vi "Test - All-In-One (SubVI).vi"(0 "START TEST":bool, 1 "STOP TEST":bool, 2 "NEXT STEP":bool, 3 "HOLD STEP":bool, 4 "Test Folder":path, 5 "Error Input":errorcluster, 7 "Test Cluster":T2={"Load Test"=0, "New Test Name"="", "Test Description"="", "Step Select"=0, "Save Test"=FALSE, "Erase Test"=FALSE, "Max Steps"=15, "Loop Limit"=5, "Continue at Loop Limit?"=FALSE, "Step N"=2, "Test Array (Standard)"=[{"Step Number"=0, "Step Description"="Step Description", "Step Time Target"=10.0, "Step Time Unit"=0, "Step End Action"=0}], "Test Array (Custom)"=[{"Custom Actions"=0, "ch0"=FALSE, "ch1"=FALSE, "ch2"=FALSE, "ch3"=FALSE}]} {"Test Array (Custom)"."Custom Actions" items=["None", "Measure Signal", "Display Plot", "Save to File"]; "Test Array (Standard)"."Step End Action" items=["Go to Next Step", "Loop to Step 0", "Loop to Step N", "Stop Test Mode", "Stop Program"]; "Test Array (Standard)"."Step Time Unit" items=["sec", "min", "hr"]; "Test Array (Standard)"."Step Time Target" min=0.01 format="%#.2f"; "Test Array (Standard)"."Step Number" min=0 step=1; "Load Test" items=["123", "a", "b", "c"]; "Step Select" step=1}, 9 "Test Cluster Ref":refnum<vi>) -> (11 "Stop Program?":bool, 13 "Test Running?":bool, 14 "Test Display":string="Mode: OFF  (Press Start to Begin)\r\r\r    ", 15 "Test Output":T1, 16 "Step Complete?":bool=TRUE, 17 "Step Number":u16, 18 "Loop Number":u16, 19 "Error Output":errorcluster)   [LabVIEW 2012]
panel:
  # "NOTE:  The only things that should need to be modified\nfor a different program are highlighted in green (on block diagram)!"
  # "9481 Relay"
  # "Custom Action"
  # "Scroll"
  # "Step"
  # "Description"
  # "Time Target"
  # "End Action"
  # "0"
  # "1"
  # "2"
  # "3"
  # "Total #\nof Steps"
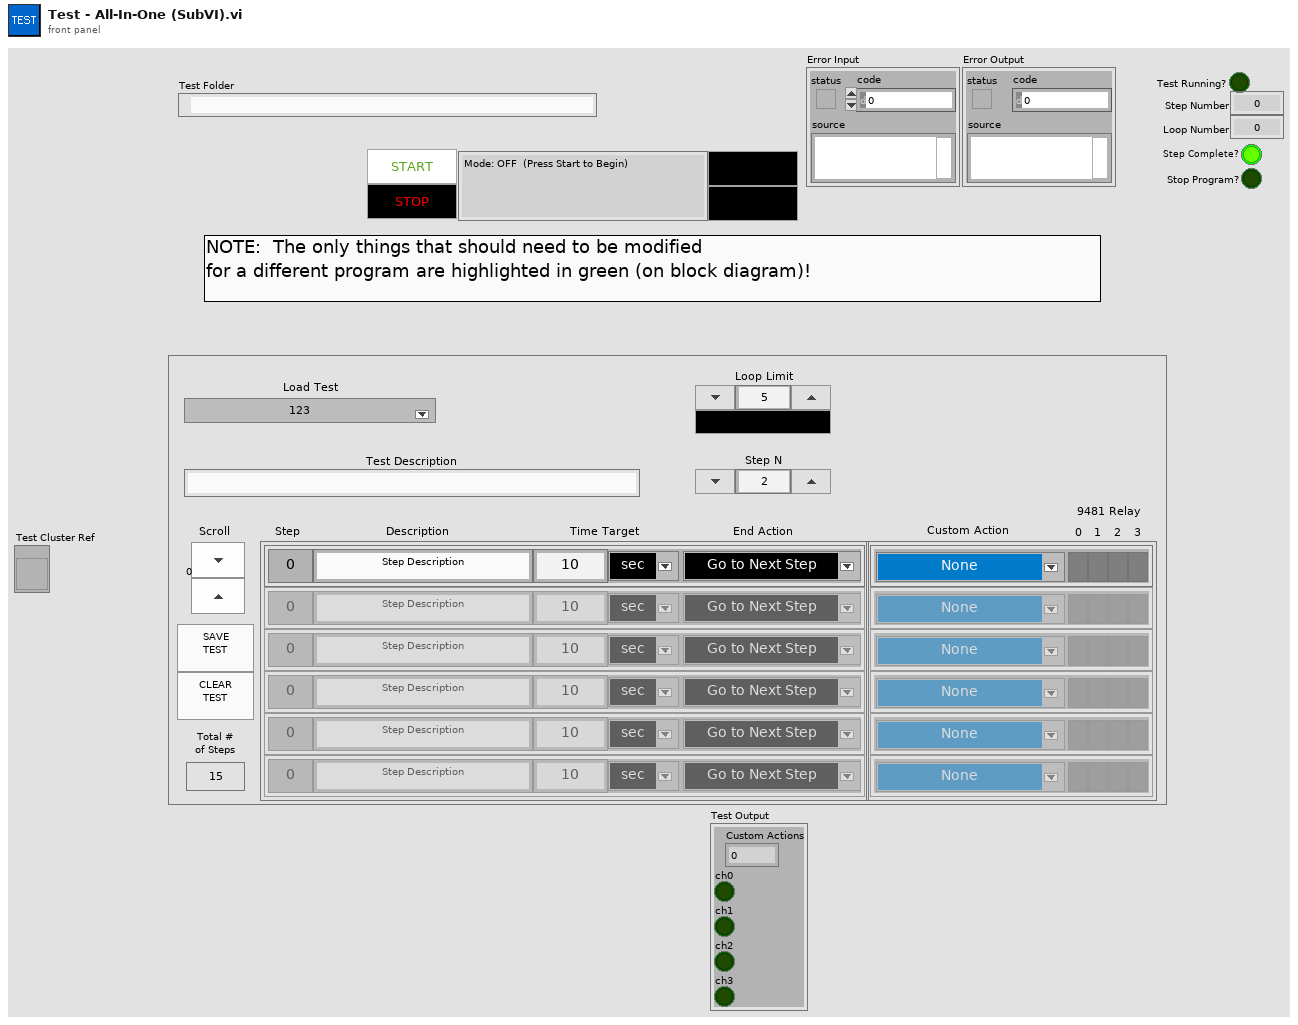
[diagram p1: front panel]
types:
  T1 = cluster{"Custom Actions":u16, "ch0":bool, "ch1":bool, "ch2":bool, "ch3":bool}
  T2 = cluster{"Load Test":u16, "New Test Name":string, "Test Description":string, "Step Select":u16, "Save Test":bool, "Erase Test":bool, "Max Steps":u16, "Loop Limit":u16, "Continue at Loop Limit?":bool, "Step N":u16, "Test Array (Standard)":cluster{"Step Number":i32, "Step Description":string, "Step Time Target":dbl, "Step Time Unit":u16, "Step End Action":u16}[], "Test Array (Custom)":cluster{"Custom Actions":u16, "ch0":bool, "ch1":bool, "ch2":bool, "ch3":bool}[]}
  T3 = cluster{"Load Test Ring":i32, "New Test Name":i32, "Test Description":i32, "Step Select":i32, "Save Test":i32, "Erase Test":i32, "Max Steps":i32, "Loop Limit":i32, "Continue at Loop Limit":i32, "Step N":i32, "Test Array (Standard)":i32, "Test Array (Custom)":i32}
  T4 = enum8{"Enabled", "Disabled", "Disabled and Grayed Out"}
  T5 = cluster{"Step Number":i32, "Step Description":string, "Step Time Target":dbl, "Step Time Unit":u16, "Step End Action":u16}[]
  T6 = cluster{"Custom Actions":u16, "ch0":bool, "ch1":bool, "ch2":bool, "ch3":bool}[]
  T7 = enum16{"open", "replace", "create", "open or create", "replace or create", "replace or create with confirmation"}
  T8 = cluster{"Step Number":i32, "Step Description":string, "Step Time Target":dbl, "Step Time Unit":u16, "Step End Action":u16}
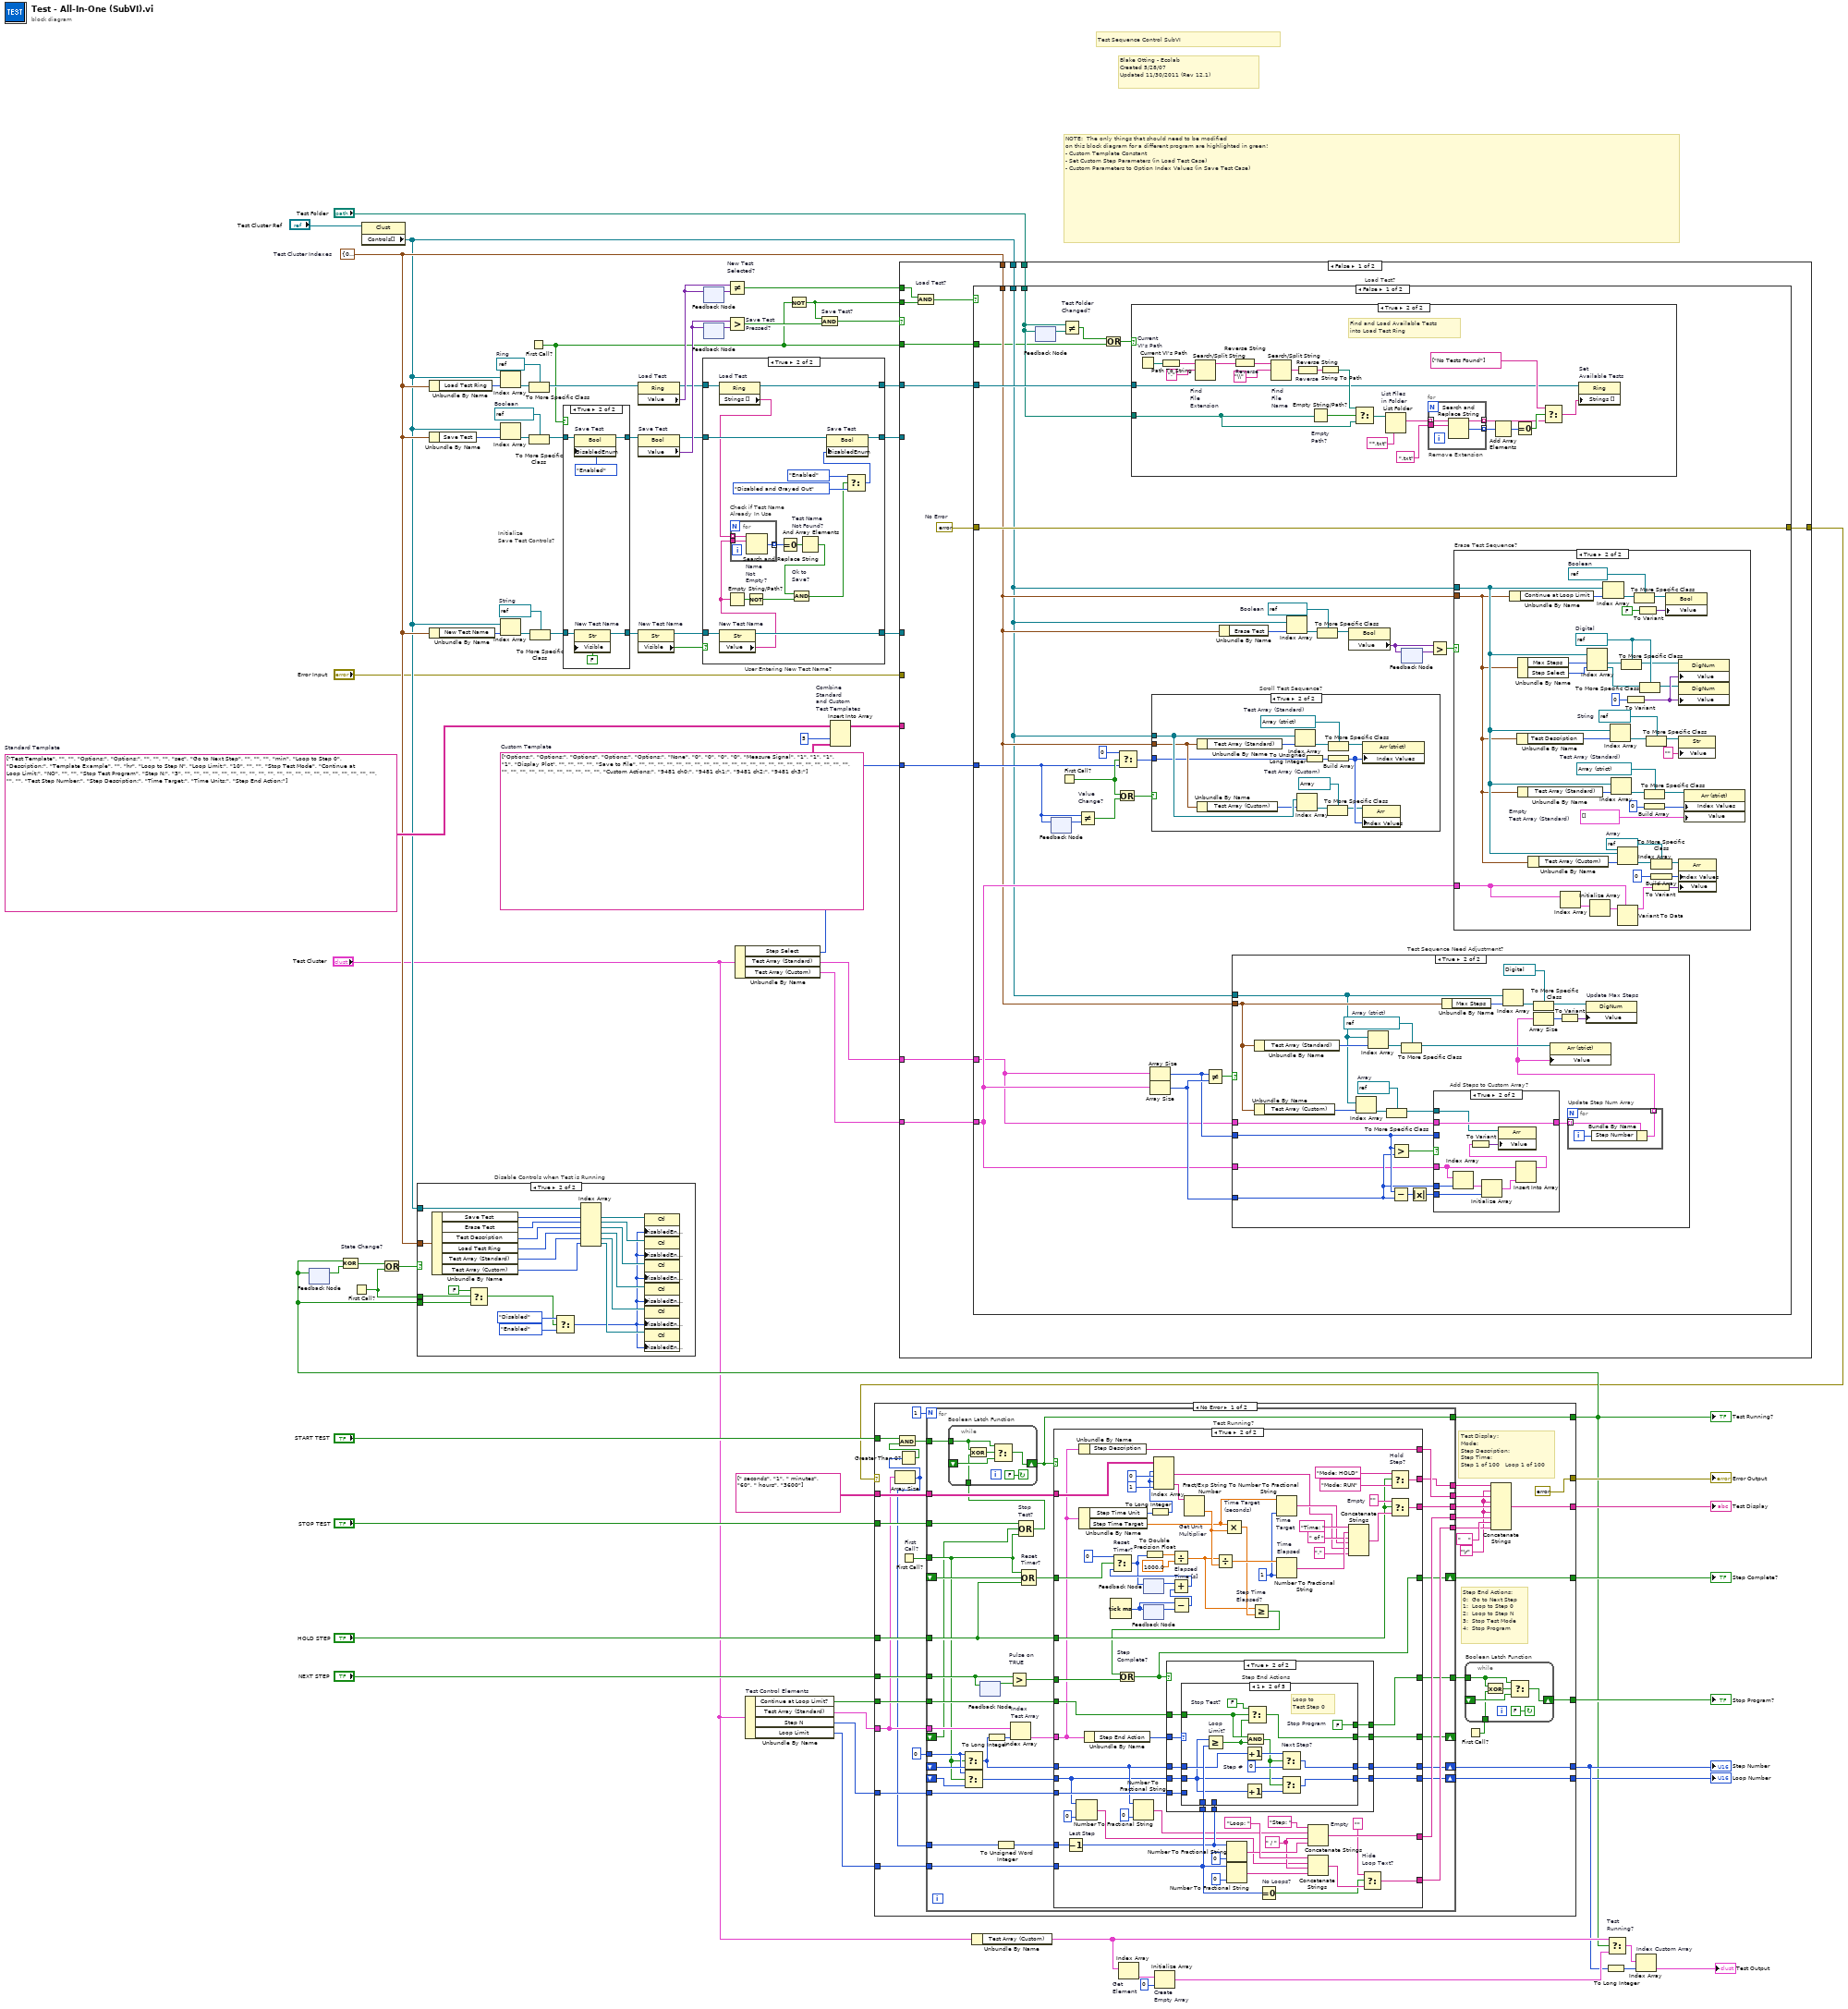
[diagram p0: block diagram]
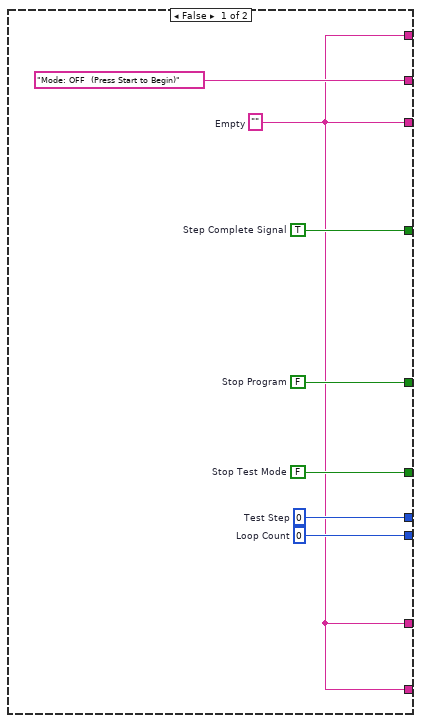
[diagram p3: hidden frame]
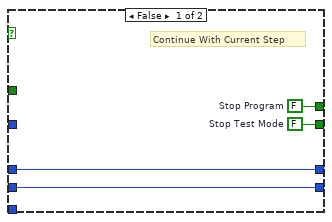
[diagram p4: hidden frame]
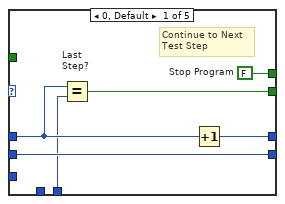
[diagram p5: hidden frame]
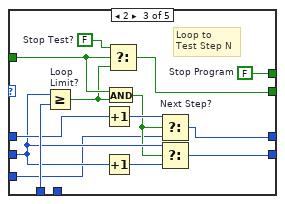
[diagram p6: hidden frame]
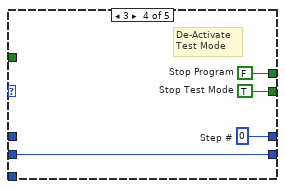
[diagram p7: hidden frame]
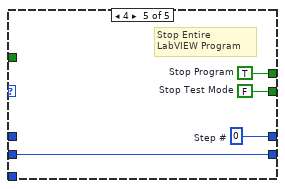
[diagram p8: hidden frame]
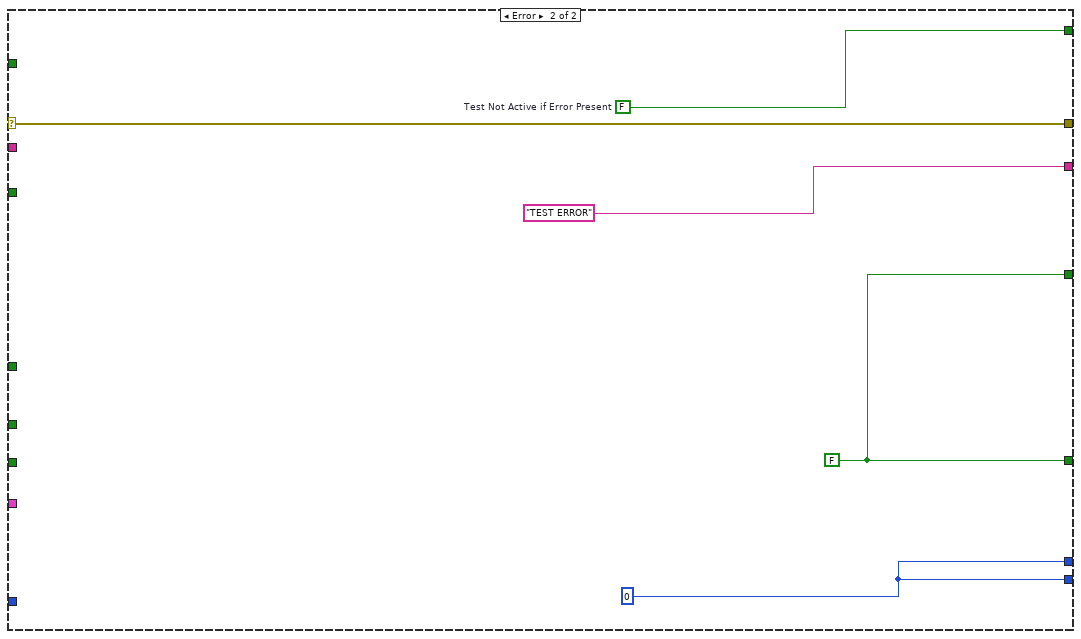
[diagram p9: hidden frame]
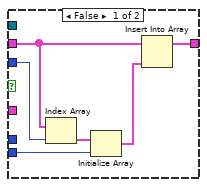
[diagram p13: hidden frame]
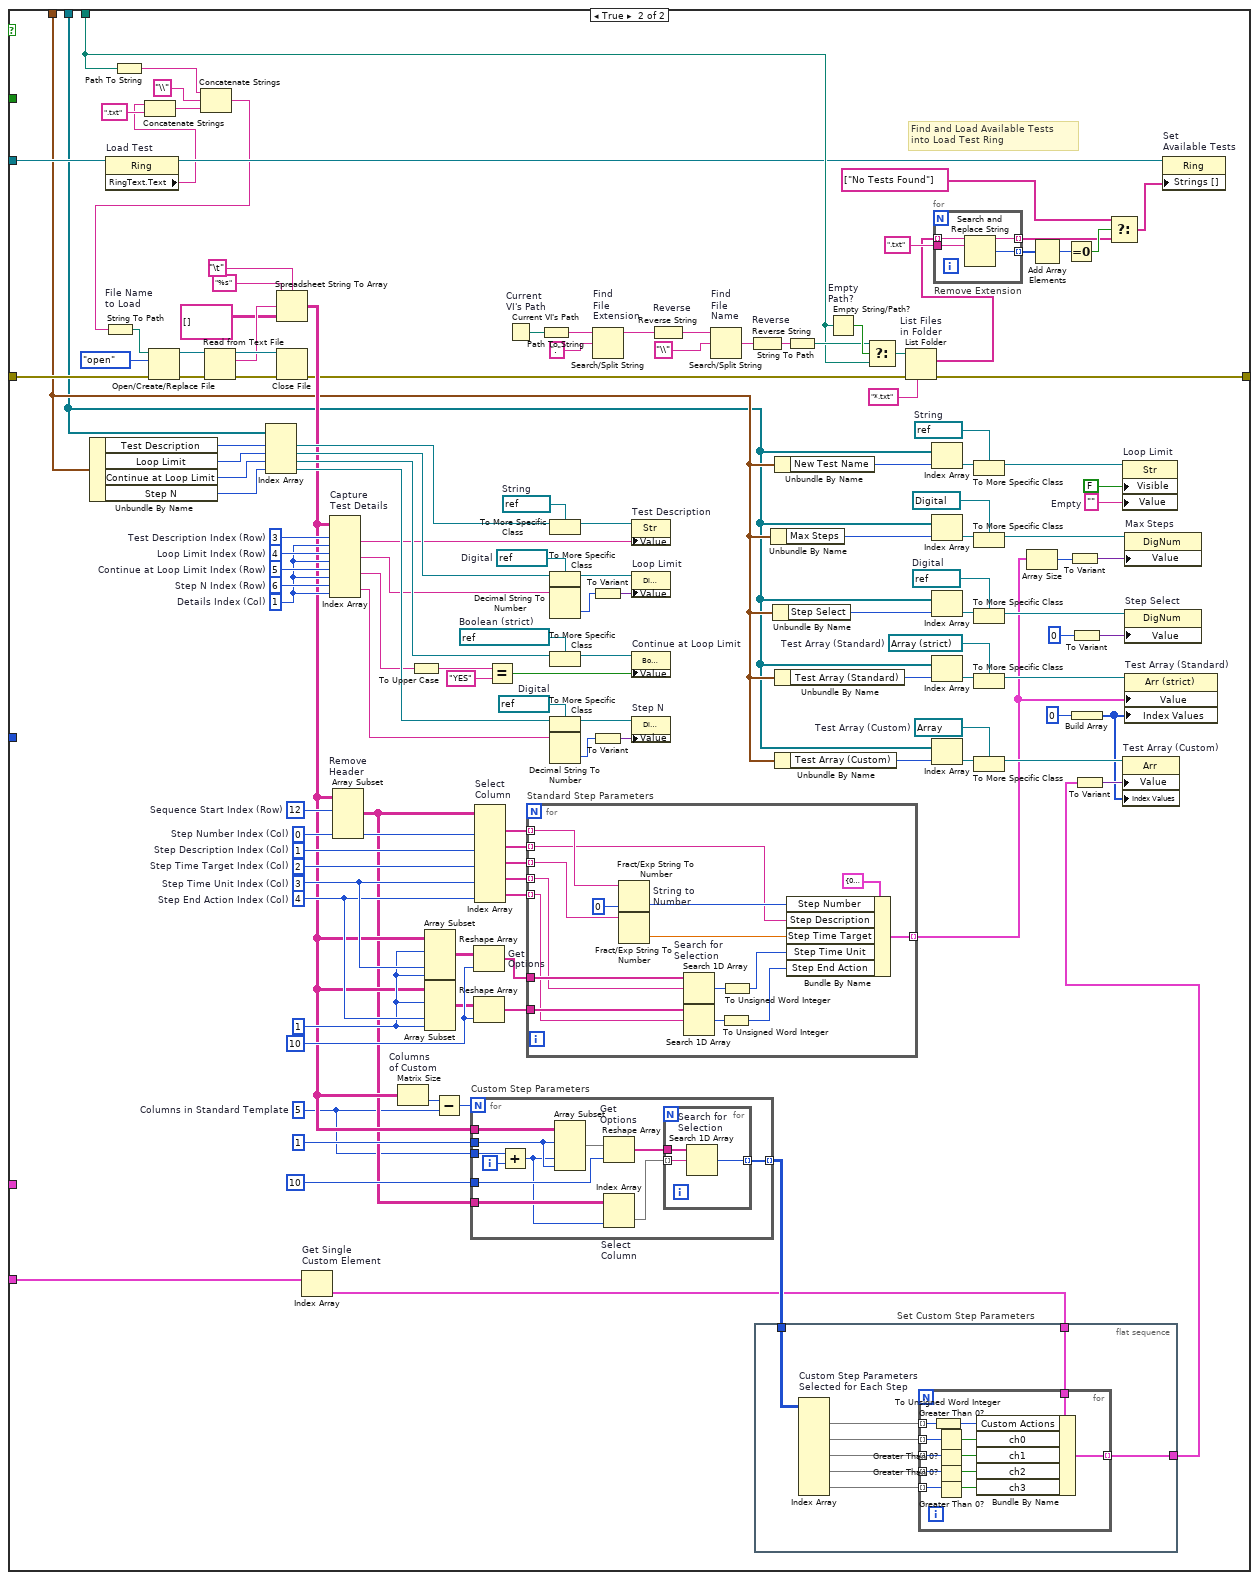
[diagram p17: hidden frame]
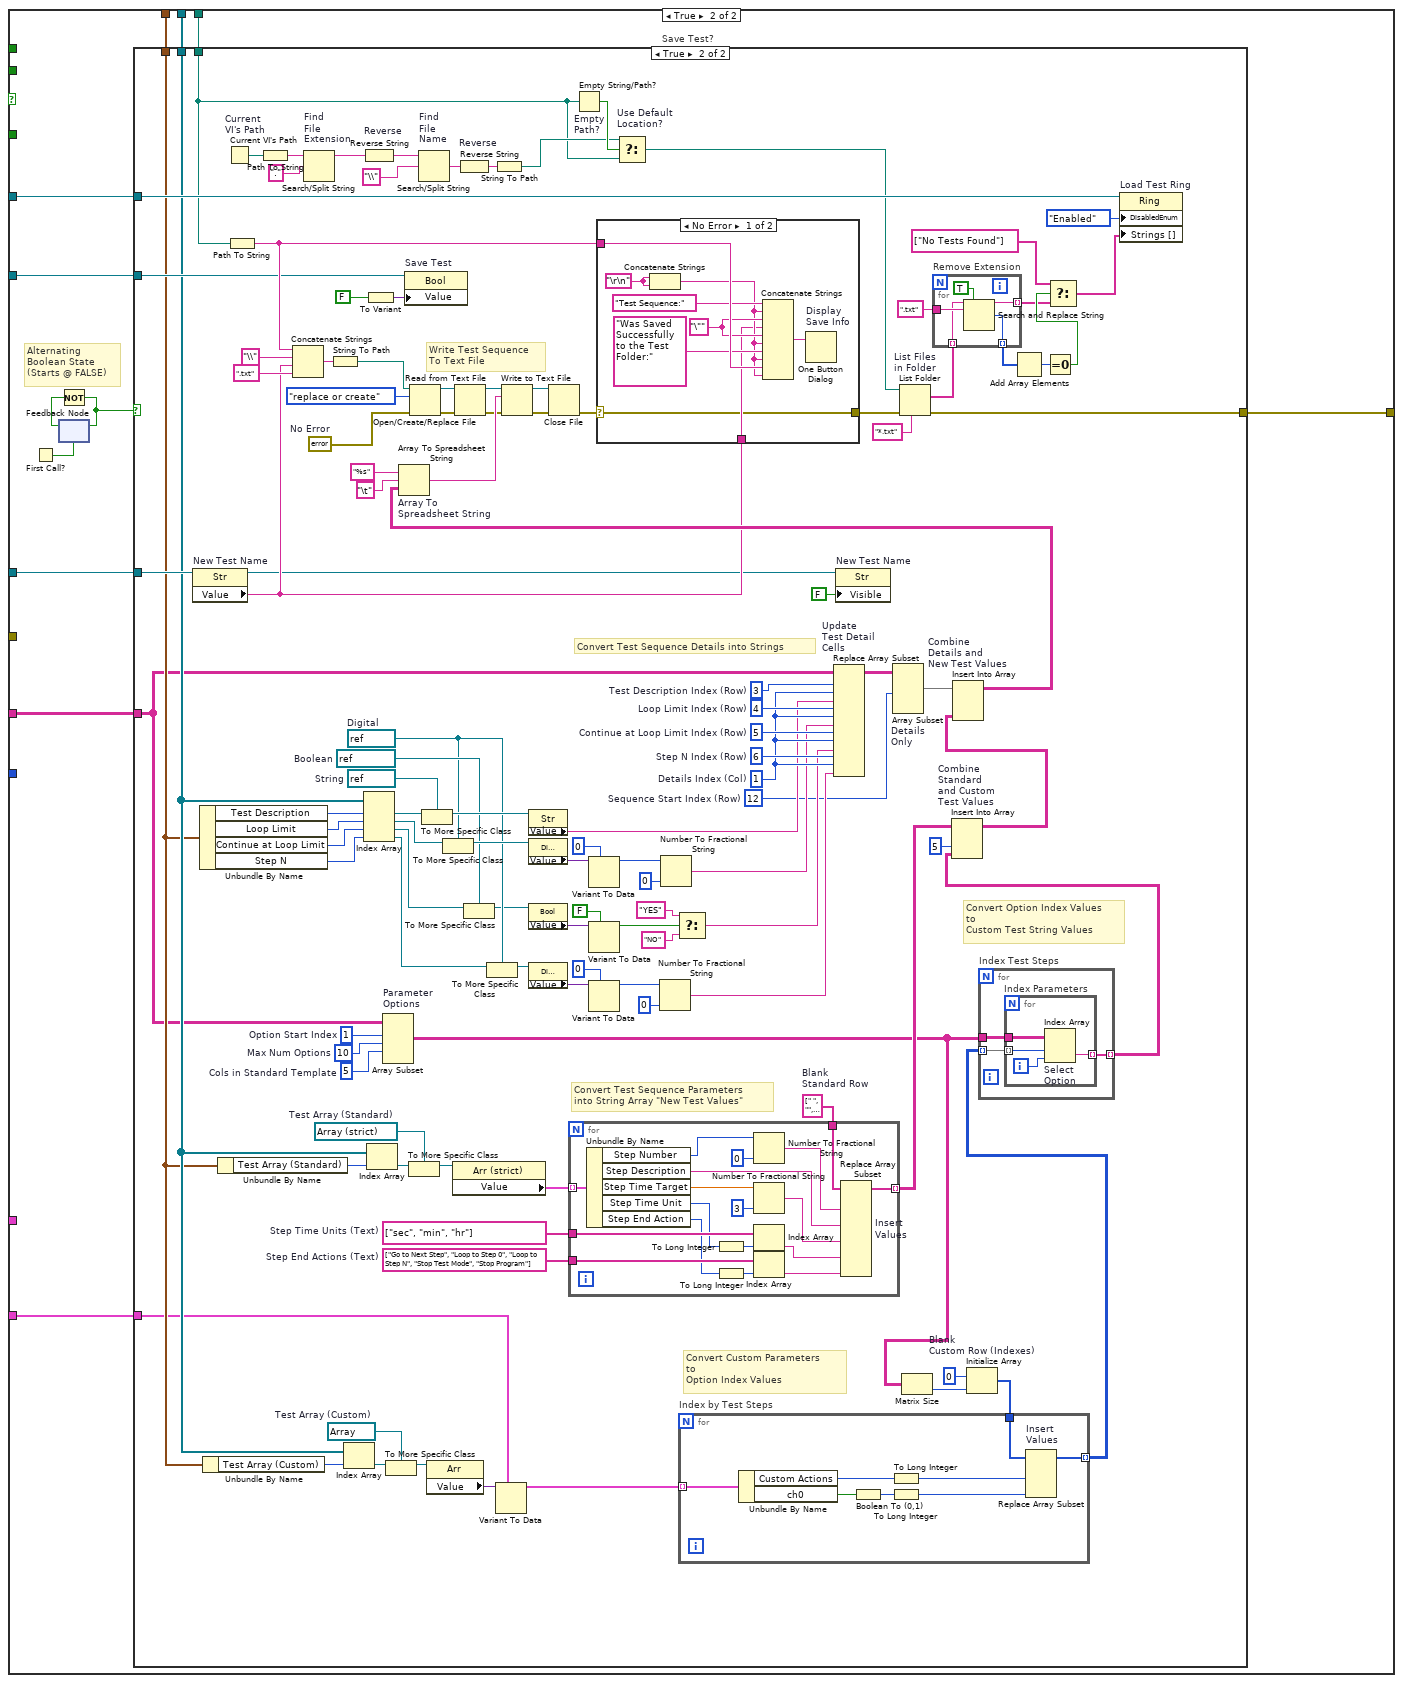
[diagram p18: hidden frame]
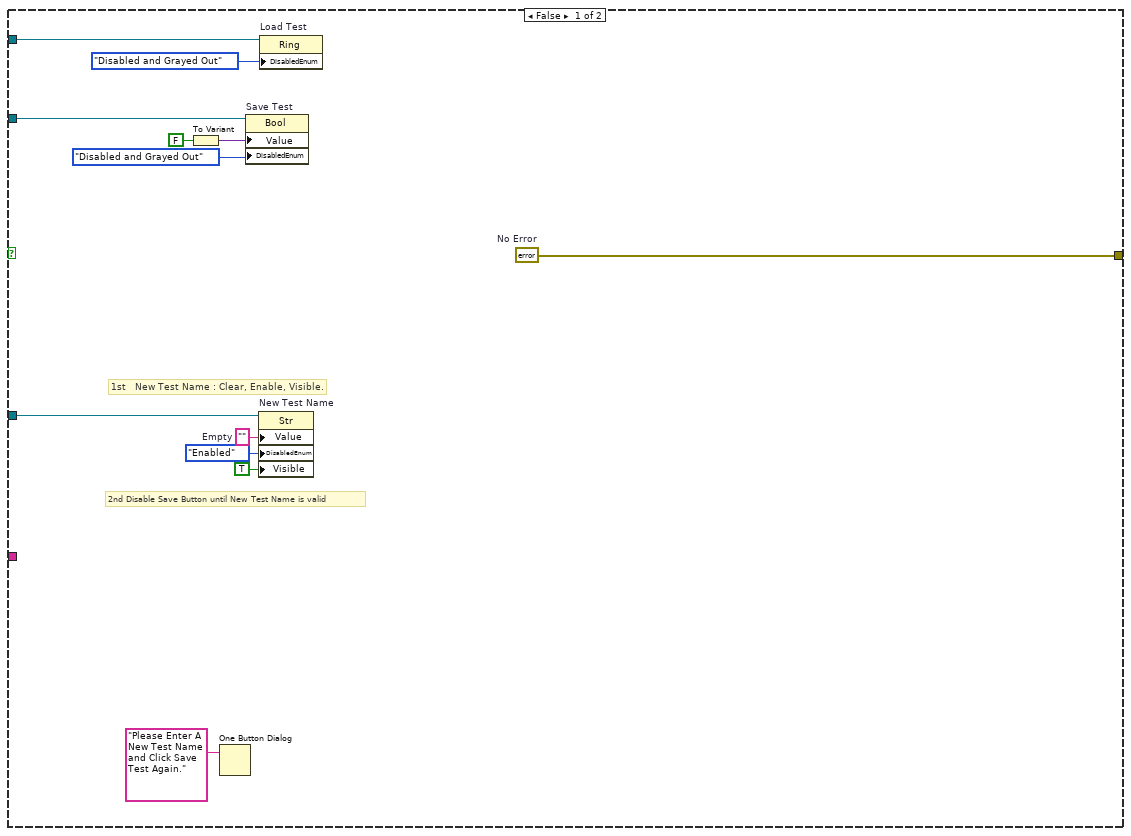
[diagram p19: hidden frame]
diagram:
  w33 = refnum<vi> refnum  # Ring
  w55 = refnum<vi> refnum  # Boolean
  w59 = refnum<vi> refnum  # String
  w64 = string[][] [["Options:", "Options:", "Options", "Options:", "Options:"], ["None", "0", "0", "0", "0"], ["Measure Signal", "1", "1", "1", "1"], ["Display Plot", "", "", "", ""], ["Save to File", "", "", "", ""], ["", "", "", "", ""], ["", "", "", "", ""], ["", "", "", "", ""], ["", "", "", "", ""], ["", "", "", "", ""], ["", "", "", "", ""], ["Custom Actions:", "9481 ch0:", "9481 ch1:", "9481 ch2:", "9481 ch3:"]]  # Custom Template
  w66 = T3 {"Load Test Ring"=0, "New Test Name"=1, "Test Description"=2, "Step Select"=3, "Save Test"=4, "Erase Test"=5, "Max Steps"=6, "Loop Limit"=7, "Continue at Loop Limit"=8, "Step N"=9, "Test Array (Standard)"=10, "Test Array (Custom)"=11}  # Test Cluster Indexes
  w71 = string[][] [["Test Template", "", "", "Options:", "Options:"], ["", "", "", "sec", "Go to Next Step"], ["", "", "", "min", "Loop to Step 0"], ["Description:", "Template Example", "", "hr", "Loop to Step N"], ["Loop Limit:", "10", "", "", "Stop Test Mode"], ["Continue at Loop Limit:", "NO", "", "", "Stop Test Program"], ["Step N:", "3", "", "", ""], ["", "", "", "", ""], ["", "", "", "", ""], ["", "", "", "", ""], ["", "", "", "", ""], ["Test Step Number:", "Step Description:", "Time Target:", "Time Units:", "Step End Action:"]]  # Standard Template
  # "NOTE:  The only things that should need to be modified\non this block diagram for a different program are highlighted in green!\n- Custom Template Constant\n- Set Custom Step Parameters (in Load Test Case)\n- Custom Parameters to Option Index Values (in Save Test Case)"
  # "Blake Otting - Ecolab\nCreated 5/28/07\nUpdated 11/30/2011 (Rev 12.1)"
  # "Test Sequence Control SubVI"
  n1 = feedback #1() -> (w30:bool)  [unwired: 1 in]
  n2 = First Call?() -> (First Call?: T/F=w27:bool)
  n3 = property class="Clust"(reference="Test Cluster Ref") -> ("Controls[]"=w65:refnum<vi>[])  [unwired: 1 in, 2 out]
  n4 = Unbundle By Name(w66) -> ("Load Test Ring"=w34:i32)
  n5 = Unbundle By Name(w66) -> ("Save Test"=w57:i32)
  n6 = Unbundle By Name(w66) -> ("New Test Name"=w61:i32)
  n7 = Index Array(array=w65, index=w34) -> (element=w32:refnum<vi>)
  n8 = Index Array(array=w65, index=w57) -> (element=w56:refnum<vi>)
  n9 = Index Array(array=w65, index=w61) -> (element=w60:refnum<vi>)
  n10 = First Call?() -> (First Call?: T/F=w8:bool)
  n11 = To More Specific Class(target class=w33, reference=w32) -> (specific class reference=w31:refnum<vi>)  [unwired: 1 in, 1 out]
  n12 = To More Specific Class(target class=w55, reference=w56) -> (specific class reference=w44:refnum<vi>)  [unwired: 1 in, 1 out]
  n13 = To More Specific Class(target class=w59, reference=w60) -> (specific class reference=w46:refnum<vi>)  [unwired: 1 in, 1 out]
  n14 = case "Initialize\nSave Test Controls?" shown="True" w8 {
    tunnel: w44 -> [w72 w79]
    tunnel: [w72 w78] -> w43
    tunnel: w46 -> [w73 w77]
    tunnel: [w73 w76] -> w45
    frame False {
    }
    frame True {
      n15 = property on="Save Test" class="Bool"(reference=w79, "DisabledEnum"=T4."Enabled" ("Disabled")) -> (reference out=w78:refnum<vi>)  [unwired: 1 in, 1 out]
      n16 = property on="New Test Name" class="Str"(reference=w77, "Visible"=FALSE) -> (reference out=w76:refnum<vi>)  [unwired: 1 in, 1 out]
    }
  }
  n17 = property on="Load Test" class="Ring"(reference=w31) -> (reference out=w39:refnum<vi>, "Value"=w40:variant)  [unwired: 1 in, 1 out]
  n18 = property on="Save Test" class="Bool"(reference=w43) -> (reference out=w49:refnum<vi>, "Value"=w53:variant)  [unwired: 1 in, 1 out]
  n19 = property on="New Test Name" class="Str"(reference=w45) -> (reference out=w51:refnum<vi>, "Visible"=w52:bool)  [unwired: 1 in, 1 out]
  n20 = case "User Entering New Test Name?" shown="True" w52 {
    tunnel: w51 -> [w82 w95]
    tunnel: w39 -> [w81 w94]
    tunnel: [w82 w90] -> w48
    tunnel: [w81 w89] -> w50
    tunnel: w49 -> [w80 w88]
    tunnel: [w80 w87] -> w47
    frame False {
    }
    frame True {
      n21 = property on="Load Test" class="Ring"(reference=w94) -> (reference out=w89:refnum<vi>, "Strings []"=w84:string[])  [unwired: 1 in, 1 out]
      n22 = property on="New Test Name" class="Str"(reference=w95) -> (reference out=w90:refnum<vi>, "Value"=w83:string)  [unwired: 1 in, 1 out]
      n23 = Empty String/Path?(string/path=w83) -> (empty?=w96:bool)
      n24 = for "Check if Test Name\nAlready In Use" {
        tunnel: w84 -> [w102] mode=indexing
        tunnel: w83 -> [w101]
        tunnel: [w100] -> w99 mode=indexing
        n25 = Search and Replace String(input string=w102, search string=w101) -> (number of replacements=w100:i32)  [unwired: 6 in, 3 out]
      }
      n26 = Not "Name\nNot\nEmpty?"(x=w96) -> (.not. x?=w91:bool)
      n27 = Equal To 0?(x=w99) -> (x = 0?=w98:bool[])
      n28 = And Array Elements "Test Name\nNot Found?"(Boolean array=w98) -> (logical AND=w97:bool)
      n29 = And "Ok to\nSave?"(x=w97, y=w91) -> (x .and. y?=w85:bool)
      n30 = Select(t=T4."Enabled" ("Disabled"), s=w85, f=T4."Disabled and Grayed Out" ("Disabled")) -> (s? t:f=w86:T4)
      n31 = property on="Save Test" class="Bool"(reference=w88, "DisabledEnum"=w86) -> (reference out=w87:refnum<vi>)  [unwired: 1 in, 1 out]
    }
  }
  n32 = feedback #2() -> (w41:variant)  [unwired: 1 in]
  n33 = feedback-in #2(w40) -> ()
  n34 = feedback #3() -> (w54:variant)  [unwired: 1 in]
  n35 = feedback-in #3(w53) -> ()
  n36 = Not Equal? "New Test\nSelected?"(x=w40, y=w41) -> (x != y?=w4:bool)
  n37 = Greater? "Save Test\nPressed?"(x=w53, y=w54) -> (0:w38:bool)
  n38 = Unbundle By Name("Test Cluster") -> ("Step Select"=w21:u16, "Test Array (Standard)"=w23:T5, "Test Array (Custom)"=w22:T6)
  n39 = Unbundle By Name "Test Control Elements"("Test Cluster") -> ("Continue at Loop Limit?"=w26:bool, "Test Array (Standard)"=w6:T5, "Step N"=w25:u16, "Loop Limit"=w24:u16)
  n40 = Not(x=w8) -> (.not. x?=w37:bool)
  n41 = And "Save Test?"(x=w37, y=w38) -> (x .and. y?=w42:bool)
  n42 = Insert Into Array "Combine\nStandard\nand Custom\nTest Templates"(array=w71, index (col)=5 ("disabled index (col)"), new element=w64) -> (w58:string[][])  [unwired: 1 in]
  n43 = case shown="False" w42 {
    tunnel: "Test Folder" -> [w111 w455]
    tunnel: w22 -> [w112 w456]
    tunnel: w58 -> [_ w457]
    tunnel: w66 -> [w114 w461]
    tunnel: w65 -> [w115 w462]
    tunnel: w47 -> [_ w460]
    tunnel: w48 -> [_ w459]
    tunnel: w50 -> [w113 w458]
    tunnel: [w106 w454] -> w7
    tunnel: "Error Input" -> [_ _]
    tunnel: w4 -> [w108 _]
    tunnel: w8 -> [w110 _]
    tunnel: w37 -> [w107 _]
    tunnel: w21 -> [w105 _]
    tunnel: w23 -> [w104 _]
    frame False {
      w103 = errorcluster {"status"=FALSE, "code"=0, "source"=""}  # No Error
      n44 = And "Load Test?"(x=w108, y=w107) -> (x .and. y?=w109:bool)
      n45 = case "Load Test?" shown="False" w109 {
        tunnel: w115 -> [w122 w267]
        tunnel: w114 -> [w123 w268]
        tunnel: w112 -> [w124 w399]
        tunnel: [w143 w276] -> w106
        tunnel: w103 -> [w143 w269]
        tunnel: w113 -> [w142 w273]
        tunnel: w110 -> [w117 _]
        tunnel: w111 -> [w119 w274]
        tunnel: w105 -> [w135 _]
        tunnel: w104 -> [w121 _]
        frame False {
          w130 = refnum<vi> refnum  # Boolean
          n46 = feedback #4() -> (w120:path)  [unwired: 1 in]
          n47 = feedback-in #4(w119) -> ()
          n48 = feedback #5() -> (w136:u16)  [unwired: 1 in]
          n49 = feedback-in #5(w135) -> ()
          n50 = First Call?() -> (First Call?: T/F=w140:bool)
          n51 = Not Equal? "Test Folder\nChanged?"(x=w119, y=w120) -> (x != y?=w118:bool)
          n52 = Not Equal? "Value\nChange?"(x=w135, y=w136) -> (x != y?=w137:bool)
          n53 = Or(x=w118, y=w117) -> (x .or. y?=w116:bool)
          n54 = Or(x=w140, y=w137) -> (x .or. y?=w138:bool)
          n55 = Select(t=u16 0 ("upper limit"), s=w140, f=w135) -> (s? t:f=w141:u16)
          n56 = case shown="True" w116 {
            tunnel: w142 -> [_ w241]
            tunnel: w119 -> [_ w240]
            frame False {
            }
            frame True {
              # "Find and Load Available Tests \ninto Load Test Ring"
              n57 = Current VI's Path "Current\nVI's Path"() -> (path=w251:path)
              n58 = Path To String(path=w251) -> (string=w256:string)
              n59 = Search/Split String "Find\nFile \nExtension"(string=w256, search string/char (-)=".") -> (substring before match=w255:string)  [unwired: 1 in, 2 out]
              n60 = Reverse String "Reverse"(1:w255) -> (0:w254:string)
              n61 = Search/Split String "Find\nFile \nName"(string=w254, search string/char (-)="\\") -> (match + rest of string=w252:string)  [unwired: 1 in, 2 out]
              n62 = Reverse String "Reverse"(1:w252) -> (0:w258:string)
              n63 = Empty String/Path? "Empty\nPath?"(string/path=w240) -> (empty?=w250:bool)
              n64 = String To Path(string=w258) -> (path=w249:path)
              n65 = Select(t=w249, s=w250, f=w240) -> (s? t:f=w259:path)
              n66 = List Folder "List Files\nin Folder"(path=w259, pattern="*.txt") -> (filenames=w261:string[])  [unwired: 1 in, 4 out]
              n67 = for "Remove Extension" {
                tunnel: w261 -> [w264] mode=indexing
                tunnel: ".txt" ("pattern") -> [w265]
                tunnel: [w263] -> w242 mode=indexing
                tunnel: [w262] -> w247 mode=indexing
                n68 = Search and Replace String(input string=w264, search string=w265) -> (result string=w263:string, number of replacements=w262:i32)  [unwired: 6 in, 2 out]
              }
              n69 = Add Array Elements(numeric array=w247) -> (sum=w246:i32)
              n70 = Equal To 0?(x=w246) -> (x = 0?=w245:bool)
              n71 = Select(t=string[] ["No Tests Found"], s=w245, f=w242) -> (s? t:f=w244:string[])
              n72 = property on="Set\nAvailable Tests" class="Ring"(reference=w241, "Strings []"=w244) -> ()  [unwired: 1 in, 2 out]
            }
          }
          n73 = Array Size(array=w121) -> (size(s)=w125:i32)
          n74 = Array Size(array=w124) -> (size(s)=w126:i32)
          n75 = case "Scroll Test Sequence?" shown="True" w138 {
            tunnel: w122 -> [_ w239]
            tunnel: w123 -> [_ w238]
            tunnel: w141 -> [_ w227]
            frame False {
            }
            frame True {
              w237 = refnum<vi> refnum  # Test Array (Custom)
              w234 = refnum<vi> refnum  # Test Array (Standard)
              n76 = Unbundle By Name(w238) -> ("Test Array (Standard)"=w235:i32)
              n77 = Unbundle By Name(w238) -> ("Test Array (Custom)"=w236:i32)
              n78 = Index Array(array=w239, index=w235) -> (element=w228:refnum<vi>)
              n79 = Index Array(array=w239, index=w236) -> (element=w231:refnum<vi>)
              n80 = To Unsigned Long Integer(number=w227) -> (unsigned 32bit integer=w230:u32)
              n81 = To More Specific Class(target class=w237, reference=w231) -> (specific class reference=w232:refnum<vi>)  [unwired: 1 in, 1 out]
              n82 = To More Specific Class(target class=w234, reference=w228) -> (specific class reference=w229:refnum<vi>)  [unwired: 1 in, 1 out]
              n83 = Build Array(w230) -> (w233:u32[])
              n84 = property class="Arr (strict)"(reference=w229, "Index Values"=w233) -> ()  [unwired: 1 in, 2 out]
              n85 = property class="Arr"(reference=w232, "Index Values"=w233) -> ()  [unwired: 1 in, 2 out]
            }
          }
          n86 = Not Equal?(x=w125, y=w126) -> (x != y?=w127:bool)
          n87 = Unbundle By Name(w123) -> ("Erase Test"=w128:i32)
          n88 = case "Test Sequence Need Adjustment?" shown="True" w127 {
            tunnel: w123 -> [_ w152]
            tunnel: w122 -> [_ w151]
            tunnel: w125 -> [_ w150]
            tunnel: w121 -> [_ w149]
            tunnel: w126 -> [_ w148]
            tunnel: w124 -> [_ w147]
            frame False {
            }
            frame True {
              w164 = refnum<vi> refnum  # Array
              w161 = refnum<vi> refnum  # Array (strict)
              n89 = Unbundle By Name(w152) -> ("Test Array (Standard)"=w162:i32)
              n90 = Unbundle By Name(w152) -> ("Test Array (Custom)"=w163:i32)
              n91 = Index Array(array=w151, index=w163) -> (element=w160:refnum<vi>)
              n92 = Index Array(array=w151, index=w162) -> (element=w159:refnum<vi>)
              n93 = To More Specific Class(target class=w164, reference=w160) -> (specific class reference=w146:refnum<vi>)  [unwired: 1 in, 1 out]
              n94 = Subtract(x=w150, y=w148) -> (x-y=w167:i32)
              n95 = Greater?(x=w150, y=w148) -> (0:w166:bool)
              n96 = To More Specific Class(target class=w161, reference=w159) -> (specific class reference=w145:refnum<vi>)  [unwired: 1 in, 1 out]
              n97 = Absolute Value(x=w167) -> (abs(x)=w168:i32)
              n98 = case "Add Steps to Custom Array?" shown="True" w166 {
                tunnel: w146 -> [_ w175]
                tunnel: w148 -> [_ w176]
                tunnel: w147 -> [_ w182]
                tunnel: w149 -> [w170 w177]
                tunnel: w168 -> [w174 w178]
                tunnel: w150 -> [w173 _]
                tunnel: [w169 w177] -> w165
                frame False {
                  n99 = Index Array(array=w170, index=w173) -> (element=w172:T8)
                  n100 = Initialize Array(w172, w174) -> (w171:T5)
                  n101 = Insert Into Array(array=w170, new element=w171) -> (w169:T5)  [unwired: 1 in]
                }
                frame True {
                  n102 = Index Array(array=w182, index=w176) -> (element=w183:T1)
                  n103 = Initialize Array(w183, w178) -> (w181:T6)
                  n104 = Insert Into Array(array=w182, new element=w181) -> (w180:T6)  [unwired: 1 in]
                  n105 = To Variant(anything=w180) -> (Variant=w179:variant)
                  n106 = property class="Arr"(reference=w175, "Value"=w179) -> ()  [unwired: 1 in, 2 out]
                }
              }
              n107 = Unbundle By Name(w152) -> ("Max Steps"=w158:i32)
              n108 = Index Array(array=w151, index=w158) -> (element=w154:refnum<vi>)
              n109 = To More Specific Class(target class=refnum<vi> refnum ("Max Steps"), reference=w154) -> (specific class reference=w157:refnum<vi>)  [unwired: 1 in, 1 out]
              n110 = for "Update Step Num Array" {
                tunnel: w165 -> [w186] mode=indexing
                tunnel: [w184] -> w144 mode=indexing
                i -> [w185]
                n111 = Bundle By Name(cluster=w186, "Step Number"=w185) -> (w184:T8)
              }
              n112 = Array Size(array=w144) -> (size(s)=w153:i32)
              n113 = property class="Arr (strict)"(reference=w145, "Value"=w144) -> ()  [unwired: 1 in, 2 out]
              n114 = To Variant(anything=w153) -> (Variant=w155:variant)
              n115 = property on="Update Max Steps" class="DigNum"(reference=w157, "Value"=w155) -> ()  [unwired: 1 in, 2 out]
            }
          }
          n116 = Index Array(array=w122, index=w128) -> (element=w129:refnum<vi>)
          n117 = To More Specific Class(target class=w130, reference=w129) -> (specific class reference=w131:refnum<vi>)  [unwired: 1 in, 1 out]
          n118 = property class="Bool"(reference=w131) -> ("Value"=w132:variant)  [unwired: 1 in, 2 out]
          n119 = feedback #6() -> (w133:variant)  [unwired: 1 in]
          n120 = feedback-in #6(w132) -> ()
          n121 = Greater?(x=w132, y=w133) -> (0:w134:bool)
          n122 = case "Erase Test Sequence?" shown="True" w134 {
            tunnel: w124 -> [_ w209]
            tunnel: w123 -> [_ w192]
            tunnel: w122 -> [_ w193]
            frame False {
            }
            frame True {
              w190 = refnum<vi> refnum  # Boolean
              w223 = refnum<vi> refnum  # Digital
              w216 = refnum<vi> refnum  # String
              w207 = refnum<vi> refnum  # Array
              w200 = T5 []  # Empty Test Array (Standard)
              w199 = refnum<vi> refnum  # Test Array (Standard)
              n123 = Unbundle By Name(w192) -> ("Continue at Loop Limit"=w191:i32)
              n124 = Unbundle By Name(w192) -> ("Test Description"=w214:i32)
              n125 = Unbundle By Name(w192) -> ("Max Steps"=w226:i32, "Step Select"=w221:i32)
              n126 = Unbundle By Name(w192) -> ("Test Array (Standard)"=w205:i32)
              n127 = Unbundle By Name(w192) -> ("Test Array (Custom)"=w206:i32)
              n128 = Index Array(array=w209) -> (element=w208:T1)  [unwired: 1 in]
              n129 = Index Array(array=w193, index #1=w226, index #2=w221) -> (element #1=w219:refnum<vi>, element #2=w222:refnum<vi>)
              n130 = Initialize Array(w208) -> (w212:T6)  [unwired: 1 in]
              n131 = Index Array(array=w193, index=w191) -> (element=w194:refnum<vi>)
              n132 = Index Array(array=w193, index=w214) -> (element=w215:refnum<vi>)
              n133 = Index Array(array=w193, index=w205) -> (element=w195:refnum<vi>)
              n134 = Index Array(array=w193, index=w206) -> (element=w201:refnum<vi>)
              n135 = Variant To Data(type=w209, Variant=w212) -> (data=w210:T6)  [unwired: 1 in, 1 out]
              n136 = To More Specific Class(target class=w223, reference=w219) -> (specific class reference=w220:refnum<vi>)  [unwired: 1 in, 1 out]
              n137 = To Variant(anything=0 ("Value")) -> (Variant=w225:variant)
              n138 = To More Specific Class(target class=w190, reference=w194) -> (specific class reference=w187:refnum<vi>)  [unwired: 1 in, 1 out]
              n139 = To Variant(anything=FALSE) -> (Variant=w189:variant)
              n140 = To More Specific Class(target class=w223, reference=w222) -> (specific class reference=w224:refnum<vi>)  [unwired: 1 in, 1 out]
              n141 = To More Specific Class(target class=w199, reference=w195) -> (specific class reference=w196:refnum<vi>)  [unwired: 1 in, 1 out]
              n142 = Build Array(u32 0 ("unsigned 32bit integer")) -> (w197:u32[])
              n143 = To More Specific Class(target class=w216, reference=w215) -> (specific class reference=w217:refnum<vi>)  [unwired: 1 in, 1 out]
              n144 = To Variant(anything=w210) -> (Variant=w211:variant)
              n145 = To More Specific Class(target class=w207, reference=w201) -> (specific class reference=w202:refnum<vi>)  [unwired: 1 in, 1 out]
              n146 = Build Array(u32 0 ("unsigned 32bit integer")) -> (w204:u32[])
              n147 = property class="Bool"(reference=w187, "Value"=w189) -> ()  [unwired: 1 in, 2 out]
              n148 = property class="DigNum"(reference=w220, "Value"=w225) -> ()  [unwired: 1 in, 2 out]
              n149 = property class="DigNum"(reference=w224, "Value"=w225) -> ()  [unwired: 1 in, 2 out]
              n150 = property class="Str"(reference=w217, "Value"="") -> ()  [unwired: 1 in, 2 out]
              n151 = property class="Arr"(reference=w202, "Index Values"=w204, "Value"=w211) -> ()  [unwired: 1 in, 2 out]
              n152 = property class="Arr (strict)"(reference=w196, "Index Values"=w197, "Value"=w200) -> ()  [unwired: 1 in, 2 out]
            }
          }
        }
        frame True {
          w300 = ""  # Empty
          w304 = refnum<vi> refnum  # String
          w309 = refnum<vi> refnum  # Digital
          w314 = refnum<vi> refnum  # Test Array (Custom)
          w322 = 5  # Columns in Standard Template
          w396 = 2  # Step Time Target Index (Col)
          w397 = 1  # Step Description Index (Col)
          w398 = 0  # Step Number Index (Col)
          w377 = refnum<vi> refnum  # Test Array (Standard)
          w374 = refnum<vi> refnum  # Digital
          w370 = refnum<vi> refnum  # Boolean (strict)
          w369 = refnum<vi> refnum  # Digital
          w355 = refnum<vi> refnum  # String
          w363 = 6  # Step N Index (Row)
          w362 = 5  # Continue at Loop Limit Index (Row)
          w361 = 4  # Loop Limit Index (Row)
          w360 = 3  # Test Description Index (Row)
          w338 = 1  # Details Index (Col)
          w394 = 4  # Step End Action Index (Col)
          w348 = 10 ("dimension size")
          w349 = 1 ("index")
          w395 = 3  # Step Time Unit Index (Col)
          w339 = 12  # Sequence Start Index (Row)
          # "Find and Load Available Tests \ninto Load Test Ring"
          n153 = Unbundle By Name(w268) -> ("Test Description"=w359:i32, "Loop Limit"=w356:i32, "Continue at Loop Limit"=w357:i32, "Step N"=w358:i32)
          n154 = property on="Load Test" class="Ring"(reference=w273) -> (reference out=w272:refnum<vi>, "RingText.Text"=w271:string)  [unwired: 1 in, 1 out]
          n155 = Path To String(path=w274) -> (string=w381:string)
          n156 = Concatenate Strings(w271, ".txt" ("string")) -> (w383:string)
          n157 = Concatenate Strings(w381, "\\" ("string"), w383) -> (w270:string)
          n158 = String To Path "File Name\nto Load"(string=w270) -> (path=w390:path)
          n159 = Open/Create/Replace File(file path (use dialog)=w390, error in=w269, operation (0:open)=T7."open") -> (refnum out=w392:refnum<file>, error out=w385:errorcluster)  [unwired: 3 in, 1 out]
          n160 = Read from Text File(file (use dialog)=w392, error in=w385) -> (refnum out=w393:refnum<file>, text=w391:string, error out=w384:errorcluster)  [unwired: 3 out]
          n161 = Index Array(array=w267, index #1=w359, index #2=w356, index #3=w357, index #4=w358) -> (element #1=w364:refnum<vi>, element #2=w365:refnum<vi>, element #3=w366:refnum<vi>, element #4=w367:refnum<vi>)
          n162 = Spreadsheet String To Array(delimiter (Tab)="\t" ("delimiter (\\t)"), format string="%s" ("format (%s)"), spreadsheet string=w391, array type (2D Dbl)=string[][] [] ("appended array")) -> (array=w325:string[][])
          n163 = Close File(refnum=w393, error in=w384) -> (error out=w277:errorcluster)  [unwired: 1 out]
          n164 = Index Array "Get Single\nCustom Element"(array=w399) -> (element=w320:T1)  [unwired: 1 in]
          n165 = Index Array "Capture\nTest Details"(array=w325, index (row) #1=w360, index (col) #1=w338, index (row) #2=w361, index (col) #2=w338, index (row) #3=w362, index (col) #3=w338, index (row) #4=w363, index (col) #4=w338) -> (element #1=w334:string, element #2=w335:string, element #3=w337:string, element #4=w336:string)
          n166 = Array Subset "Remove\nHeader"(array=w325, index (row)=w339) -> (w324:string[][])  [unwired: 3 in]
          n167 = Matrix Size "Columns\nof Custom"(0:w325) -> (2:w328:i32)  [unwired: 1 out]
          n168 = To Upper Case(1:w337) -> (0:w372:string)
          n169 = Array Subset(array=w325, index (row)=w349, index (col)=w395, length (col)=w349) -> (w345:string[][])  [unwired: 1 in]
          n170 = Array Subset(array=w325, index (row)=w349, index (col)=w394, length (col)=w349) -> (w347:string[][])  [unwired: 1 in]
          n171 = Subtract(x=w328, y=w322) -> (x-y=w323:i32)
          n172 = for "Custom Step Parameters" {
            N: w323 -> [_]
            tunnel: 1 ("index") -> [w433]
            tunnel: 10 ("dimension size") -> [w432]
            tunnel: w325 -> [w431]
            tunnel: w324 -> [w430]
            tunnel: w322 -> [w428]
            tunnel: [w424] -> w321 mode=indexing
            i -> [w429]
            n173 = Add(x=w428, y=w429) -> (x+y=w427:i32)
            n174 = Array Subset(array=w431, index (row)=w433, index (col)=w427, length (col)=w433) -> (w434:string[][])  [unwired: 1 in]
            n175 = Reshape Array "Get\nOptions"(w434, w432) -> (w425:string[])
            n176 = Index Array "Select\nColumn"(array=w430, index (col)=w427) -> (element=w426:string[])  [unwired: 1 in]
            n177 = for {
              tunnel: w426 -> [w436] mode=indexing
              tunnel: w425 -> [w437]
              tunnel: [w435] -> w424 mode=indexing
              n178 = Search 1D Array "Search for\nSelection"(1D array=w437, element=w436) -> (index of element=w435:i32)  [unwired: 1 in]
            }
          }
          n179 = Reshape Array "Get\nOptions"(w345, w348) -> (w346:string[])
          n180 = Reshape Array(w347, w348) -> (w350:string[])
          n181 = Index Array "Select\nColumn"(array=w324, index (col) #1=w398, index (col) #2=w397, index (col) #3=w396, index (col) #4=w395, index (col) #5=w394) -> (element #1=w340:string[], element #2=w341:string[], element #3=w342:string[], element #4=w343:string[], element #5=w344:string[])  [unwired: 5 in]
          n182 = Equal?(x=w372, y="YES") -> (x = y?=w373:bool)
          n183 = Current VI's Path "Current\nVI's Path"() -> (path=w287:path)
          n184 = for "Standard Step Parameters" {
            tunnel: w340 -> [w452] mode=indexing
            tunnel: w341 -> [w449] mode=indexing
            tunnel: w342 -> [w447] mode=indexing
            tunnel: w343 -> [w443] mode=indexing
            tunnel: w344 -> [w439] mode=indexing
            tunnel: [w446] -> w297 mode=indexing
            tunnel: w346 -> [w444]
            tunnel: w350 -> [w440]
            n185 = Fract/Exp String To Number "String to\nNumber"(string=w452, default (0 dbl)=0) -> (number=w450:i32)  [unwired: 2 in, 1 out]
            n186 = Fract/Exp String To Number ("String to\nNumber")(string=w447) -> (number=w448:dbl)  [unwired: 3 in, 1 out]
            n187 = Search 1D Array "Search for\nSelection"(1D array=w444, element=w443) -> (index of element=w445:i32)  [unwired: 1 in]
            n188 = Search 1D Array(1D array=w440, element=w439) -> (index of element=w441:i32)  [unwired: 1 in]
            n189 = To Unsigned Word Integer(number=w441) -> (unsigned 16bit integer=w438:u16)
            n190 = To Unsigned Word Integer(number=w445) -> (unsigned 16bit integer=w442:u16)
            n191 = Bundle By Name(cluster=T8 {"Step Number"=0, "Step Description"="", "Step Time Target"=0.0, "Step Time Unit"=0, "Step End Action"=0} ("Standard Test Step Parameters"), "Step Number"=w450, "Step Description"=w449, "Step Time Target"=w448, "Step Time Unit"=w442, "Step End Action"=w438) -> (w446:T8)
          }
          n192 = Path To String(path=w287) -> (string=w292:string)
          n193 = To More Specific Class(target class=w355, reference=w364) -> (specific class reference=w351:refnum<vi>)  [unwired: 1 in, 1 out]
          n194 = To More Specific Class(target class=w369, reference=w365) -> (specific class reference=w352:refnum<vi>)  [unwired: 1 in, 1 out]
          n195 = Decimal String To Number(string=w335) -> (number=w368:i32)  [unwired: 2 in, 1 out]
          n196 = To More Specific Class(target class=w370, reference=w366) -> (specific class reference=w353:refnum<vi>)  [unwired: 1 in, 1 out]
          n197 = To More Specific Class(target class=w374, reference=w367) -> (specific class reference=w354:refnum<vi>)  [unwired: 1 in, 1 out]
          n198 = Decimal String To Number(string=w336) -> (number=w312:i32)  [unwired: 2 in, 1 out]
          n199 = Search/Split String "Find\nFile \nExtension"(string=w292, search string/char (-)=".") -> (substring before match=w291:string)  [unwired: 1 in, 2 out]
          n200 = To Variant(anything=w368) -> (Variant=w313:variant)
          n201 = To Variant(anything=w312) -> (Variant=w311:variant)
          n202 = property on="Test Description" class="Str"(reference=w351, "Value"=w334) -> ()  [unwired: 1 in, 2 out]
          n203 = property on="Loop Limit" class="DigNum"(reference=w352, "Value"=w313) -> ()  [unwired: 1 in, 2 out]
          n204 = property on="Continue at Loop Limit" class="Bool (strict)"(reference=w353, "Value"=w373) -> ()  [unwired: 1 in, 2 out]
          n205 = property on="Step N" class="DigNum"(reference=w354, "Value"=w311) -> ()  [unwired: 1 in, 2 out]
          n206 = Reverse String "Reverse"(1:w291) -> (0:w290:string)
          n207 = Search/Split String "Find\nFile \nName"(string=w290, search string/char (-)="\\") -> (match + rest of string=w288:string)  [unwired: 1 in, 2 out]
          n208 = Reverse String "Reverse"(1:w288) -> (0:w294:string)
          n209 = flat-sequence "Set Custom Step Parameters" {
            tunnel: w321 -> [w411]
            tunnel: w320 -> [w408]
            tunnel: [w407] -> w318
            frame #0 {
              n210 = Index Array "Custom Step Parameters\nSelected for Each Step"(array=w411) -> (element #1=w410:i32[], element #2=w409:i32[], element #3=w406:i32[], element #4=w405:i32[], element #5=w404:i32[])  [unwired: 10 in]
              n211 = for {
                tunnel: w410 -> [w421] mode=indexing
                tunnel: w409 -> [w420] mode=indexing
                tunnel: w408 -> [w419]
                tunnel: [w418] -> w407 mode=indexing
                tunnel: w406 -> [w417] mode=indexing
                tunnel: w405 -> [w413] mode=indexing
                tunnel: w404 -> [w412] mode=indexing
                n212 = To Unsigned Word Integer(number=w421) -> (unsigned 16bit integer=w423:u16)
                n213 = Greater Than 0?(x=w420) -> (x > 0?=w422:bool)
                n214 = Greater Than 0?(x=w417) -> (x > 0?=w416:bool)
                n215 = Greater Than 0?(x=w413) -> (x > 0?=w415:bool)
                n216 = Greater Than 0?(x=w412) -> (x > 0?=w414:bool)
                n217 = Bundle By Name(cluster=w419, "Custom Actions"=w423, "ch0"=w422, "ch1"=w416, "ch2"=w415, "ch3"=w414) -> (w418:T1)
              }
            }
          }
          n218 = Unbundle By Name(w268) -> ("Max Steps"=w379:i32)
          n219 = Unbundle By Name(w268) -> ("Step Select"=w310:i32)
          n220 = Unbundle By Name(w268) -> ("New Test Name"=w303:i32)
          n221 = Unbundle By Name(w268) -> ("Test Array (Standard)"=w375:i32)
          n222 = Unbundle By Name(w268) -> ("Test Array (Custom)"=w316:i32)
          n223 = String To Path(string=w294) -> (path=w285:path)
          n224 = Empty String/Path? "Empty\nPath?"(string/path=w274) -> (empty?=w286:bool)
          n225 = Select(t=w285, s=w286, f=w274) -> (s? t:f=w295:path)
          n226 = List Folder "List Files\nin Folder"(path=w295, pattern="*.txt", error in=w277) -> (filenames=w266:string[], error out=w276:errorcluster)  [unwired: 3 out]
          n227 = Index Array(array=w267, index=w303) -> (element=w302:refnum<vi>)
          n228 = Index Array(array=w267, index=w379) -> (element=w331:refnum<vi>)
          n229 = Index Array(array=w267, index=w310) -> (element=w306:refnum<vi>)
          n230 = Index Array(array=w267, index=w375) -> (element=w376:refnum<vi>)
          n231 = Index Array(array=w267, index=w316) -> (element=w315:refnum<vi>)
          n232 = for "Remove Extension" {
            tunnel: w266 -> [w402] mode=indexing
            tunnel: ".txt" ("pattern") -> [w403]
            tunnel: [w401] -> w278 mode=indexing
            tunnel: [w400] -> w283 mode=indexing
            n233 = Search and Replace String(input string=w402, search string=w403) -> (result string=w401:string, number of replacements=w400:i32)  [unwired: 6 in, 2 out]
          }
          n234 = To More Specific Class(target class=w304, reference=w302) -> (specific class reference=w301:refnum<vi>)  [unwired: 1 in, 1 out]
          n235 = To More Specific Class(target class=refnum<vi> refnum ("Max Steps"), reference=w331) -> (specific class reference=w333:refnum<vi>)  [unwired: 1 in, 1 out]
          n236 = To More Specific Class(target class=w309, reference=w306) -> (specific class reference=w307:refnum<vi>)  [unwired: 1 in, 1 out]
          n237 = To More Specific Class(target class=w377, reference=w376) -> (specific class reference=w378:refnum<vi>)  [unwired: 1 in, 1 out]
          n238 = To More Specific Class(target class=w314, reference=w315) -> (specific class reference=w317:refnum<vi>)  [unwired: 1 in, 1 out]
          n239 = Array Size(array=w297) -> (size(s)=w329:i32)
          n240 = Add Array Elements(numeric array=w283) -> (sum=w282:i32)
          n241 = Equal To 0?(x=w282) -> (x = 0?=w281:bool)
          n242 = To Variant(anything=w329) -> (Variant=w330:variant)
          n243 = To Variant(anything=u32 0) -> (Variant=w308:variant)
          n244 = Build Array(u32 0) -> (w298:u32[])
          n245 = To Variant(anything=w318) -> (Variant=w319:variant)
          n246 = Select(t=string[] ["No Tests Found"], s=w281, f=w278) -> (s? t:f=w280:string[])
          n247 = property on="Loop Limit" class="Str"(reference=w301, "Visible"=FALSE, "Value"=w300) -> ()  [unwired: 1 in, 2 out]
          n248 = property on="Test Array (Custom)" class="Arr"(reference=w317, "Value"=w319, "Index Values"=w298) -> ()  [unwired: 1 in, 2 out]
          n249 = property on="Max Steps" class="DigNum"(reference=w333, "Value"=w330) -> ()  [unwired: 1 in, 2 out]
          n250 = property on="Step Select" class="DigNum"(reference=w307, "Value"=w308) -> ()  [unwired: 1 in, 2 out]
          n251 = property on="Test Array (Standard)" class="Arr (strict)"(reference=w378, "Value"=w297, "Index Values"=w298) -> ()  [unwired: 1 in, 2 out]
          n252 = property on="Set\nAvailable Tests" class="Ring"(reference=w272, "Strings []"=w280) -> ()  [unwired: 1 in, 2 out]
        }
      }
    }
    frame True {
      # "Alternating\nBoolean State\n(Starts @ FALSE)"
      n253 = First Call?() -> (First Call?: T/F=w464:bool)
      n254 = feedback #7(w464) -> (w465:bool)
      n255 = Not(x=w465) -> (.not. x?=w463:bool)
      n256 = feedback-in #7(w463) -> ()
      n257 = case "Save Test?" shown="True" w463 {
        tunnel: w461 -> [_ w497]
        tunnel: w462 -> [_ w498]
        tunnel: w460 -> [w473 w527]
        tunnel: w459 -> [w470 w531]
        tunnel: w458 -> [w469 w526]
        tunnel: w457 -> [_ w490]
        tunnel: w456 -> [_ w489]
        tunnel: w455 -> [_ w502]
        tunnel: [w466 w503] -> w454
        frame False {
          w466 = errorcluster {"status"=FALSE, "code"=0, "source"=""}  # No Error
          w475 = ""  # Empty
          # "2nd Disable Save Button until New Test Name is valid"
          # "1st   New Test Name : Clear, Enable, Visible."
          n258 = To Variant(anything=FALSE ("Value")) -> (Variant=w471:variant)
          n259 = One Button Dialog(message="Please Enter A New Test Name and Click Save Test Again.") -> ()  [unwired: 1 in, 1 out]
          n260 = property on="Save Test" class="Bool"(reference=w473, "Value"=w471, "DisabledEnum"=T4."Disabled and Grayed Out" ("Disabled")) -> ()  [unwired: 1 in, 2 out]
          n261 = property on="New Test Name" class="Str"(reference=w470, "Value"=w475, "DisabledEnum"=T4."Enabled" ("Disabled"), "Visible"=TRUE) -> ()  [unwired: 1 in, 2 out]
          n262 = property on="Load Test" class="Ring"(reference=w469, "DisabledEnum"=T4."Disabled and Grayed Out" ("Disabled")) -> ()  [unwired: 1 in, 2 out]
        }
        frame True {
          w483 = string[] [" ", "", "", "", " "]  # Blank Standard Row
          w485 = errorcluster {"status"=FALSE, "code"=0, "source"=""}  # No Error
          w492 = 5  # Cols in Standard Template
          w494 = 1  # Option Start Index
          w493 = 10  # Max Num Options
          w499 = refnum<vi> refnum  # Test Array (Custom)
          w540 = refnum<vi> refnum  # Digital
          w558 = refnum<vi> refnum  # Boolean
          w549 = 12  # Sequence Start Index (Row)
          w569 = string[] ["sec", "min", "hr"]  # Step Time Units (Text)
          w568 = string[] ["Go to Next Step", "Loop to Step 0", "Loop to Step N", "Stop Test Mode", "Stop Program"]  # Step End Actions (Text)
          w570 = refnum<vi> refnum  # Test Array (Standard)
          w586 = refnum<vi> refnum  # String
          w594 = 6  # Step N Index (Row)
          w597 = 5  # Continue at Loop Limit Index (Row)
          w595 = 4  # Loop Limit Index (Row)
          w596 = 3  # Test Description Index (Row)
          w593 = 1  # Details Index (Col)
          # "Convert Custom Parameters\nto\nOption Index Values"
          # "Convert Option Index Values\nto\nCustom Test String Values"
          # "Write Test Sequence\nTo Text File"
          # "Convert Test Sequence Details into Strings"
          # "Convert Test Sequence Parameters\ninto String Array \"New Test Values\""
          n263 = property on="New Test Name" class="Str"(reference=w531) -> (reference out=w530:refnum<vi>, "Value"=w532:string)  [unwired: 1 in, 1 out]
          n264 = Unbundle By Name(w497) -> ("Test Description"=w581:i32, "Loop Limit"=w584:i32, "Continue at Loop Limit"=w583:i32, "Step N"=w582:i32)
          n265 = Unbundle By Name(w497) -> ("Test Array (Custom)"=w500:i32)
          n266 = Unbundle By Name(w497) -> ("Test Array (Standard)"=w573:i32)
          n267 = Current VI's Path "Current\nVI's Path"() -> (path=w515:path)
          n268 = Path To String(path=w502) -> (string=w559:string)
          n269 = Path To String(path=w515) -> (string=w520:string)
          n270 = Concatenate Strings(w559, "\\" ("string"), w532, ".txt" ("string")) -> (w578:string)
          n271 = Search/Split String "Find\nFile \nExtension"(string=w520, search string/char (-)=".") -> (substring before match=w519:string)  [unwired: 1 in, 2 out]
          n272 = String To Path(string=w578) -> (path=w574:path)
          n273 = Index Array(array=w498, index=w500) -> (element=w496:refnum<vi>)
          n274 = Reverse String "Reverse"(1:w519) -> (0:w518:string)
          n275 = Index Array(array=w498, index #1=w581, index #2=w584, index #3=w583, index #4=w582) -> (element #1=w592:refnum<vi>, element #2=w589:refnum<vi>, element #3=w557:refnum<vi>, element #4=w585:refnum<vi>)
          n276 = To Variant(anything=FALSE ("Value")) -> (Variant=w528:variant)
          n277 = Index Array(array=w498, index=w573) -> (element=w572:refnum<vi>)
          n278 = Array Subset "Parameter\nOptions"(array=w490, index (row)=w494, length (row)=w493, index (col)=w492) -> (w479:string[][])  [unwired: 1 in]
          n279 = To More Specific Class(target class=w499, reference=w496) -> (specific class reference=w495:refnum<vi>)  [unwired: 1 in, 1 out]
          n280 = property on="Save Test" class="Bool"(reference=w527, "Value"=w528) -> ()  [unwired: 1 in, 2 out]
          n281 = To More Specific Class(target class=w570, reference=w572) -> (specific class reference=w571:refnum<vi>)  [unwired: 1 in, 1 out]
          n282 = Open/Create/Replace File(file path (use dialog)=w574, error in=w485, operation (0:open)=T7."replace or create") -> (refnum out=w575:refnum<file>, error out=w577:errorcluster)  [unwired: 3 in, 1 out]
          n283 = Search/Split String "Find\nFile \nName"(string=w518, search string/char (-)="\\") -> (match + rest of string=w516:string)  [unwired: 1 in, 2 out]
          n284 = To More Specific Class(target class=w586, reference=w592) -> (specific class reference=w591:refnum<vi>)  [unwired: 1 in, 1 out]
          n285 = property class="Arr"(reference=w495) -> ("Value"=w488:variant)  [unwired: 1 in, 2 out]
          n286 = To More Specific Class(target class=w540, reference=w589) -> (specific class reference=w588:refnum<vi>)  [unwired: 1 in, 1 out]
          n287 = property class="Arr (strict)"(reference=w571) -> ("Value"=w484:T5)  [unwired: 1 in, 2 out]
          n288 = Read from Text File(file (use dialog)=w575, error in=w577) -> (refnum out=w561:refnum<file>, error out=w560:errorcluster)  [unwired: 4 out]
          n289 = Reverse String "Reverse"(1:w516) -> (0:w522:string)
          n290 = To More Specific Class(target class=w558, reference=w557) -> (specific class reference=w536:refnum<vi>)  [unwired: 1 in, 1 out]
          n291 = To More Specific Class(target class=w540, reference=w585) -> (specific class reference=w587:refnum<vi>)  [unwired: 1 in, 1 out]
          n292 = String To Path(string=w522) -> (path=w513:path)
          n293 = Variant To Data(type=w489, Variant=w488) -> (data=w482:T6)  [unwired: 1 in, 1 out]
          n294 = property class="Str"(reference=w591) -> ("Value"=w590:string)  [unwired: 1 in, 2 out]
          n295 = property class="DigNum"(reference=w588) -> ("Value"=w542:variant)  [unwired: 1 in, 2 out]
          n296 = property class="Bool"(reference=w536) -> ("Value"=w535:variant)  [unwired: 1 in, 2 out]
          n297 = property class="DigNum"(reference=w587) -> ("Value"=w539:variant)  [unwired: 1 in, 2 out]
          n298 = for {
            tunnel: w484 -> [w645] mode=indexing
            tunnel: w569 -> [w640]
            tunnel: w568 -> [w639]
            tunnel: [w631] -> w486 mode=indexing
            tunnel: w483 -> [w628]
            n299 = Unbundle By Name(w645) -> ("Step Number"=w635:i32, "Step Description"=w633:string, "Step Time Target"=w641:dbl, "Step Time Unit"=w638:u16, "Step End Action"=w637:u16)
            n300 = To Long Integer(number=w638) -> (32bit integer=w643:i32)
            n301 = To Long Integer(number=w637) -> (32bit integer=w644:i32)
            n302 = Number To Fractional String(number=w635, precision (6)=i16 0) -> (F-format string=w634:string)  [unwired: 2 in]
            n303 = Number To Fractional String(number=w641, precision (6)=i16 3) -> (F-format string=w632:string)  [unwired: 2 in]
            n304 = Index Array(array=w640, index=w643) -> (element=w630:string)
            n305 = Index Array(array=w639, index=w644) -> (element=w629:string)
            n306 = Replace Array Subset "Insert\nValues"(array=w628, new element #1=w634, new element #2=w633, new element #3=w632, new element #4=w630, new element #5=w629) -> (w631:string[])  [unwired: 5 in]
          }
          n307 = Empty String/Path? "Empty\nPath?"(string/path=w502) -> (empty?=w514:bool)
          n308 = Variant To Data(type=u16 0, Variant=w542) -> (data=w541:u16)  [unwired: 1 in, 1 out]
          n309 = Variant To Data(type=FALSE, Variant=w535) -> (data=w533:bool)  [unwired: 1 in, 1 out]
          n310 = Variant To Data(type=u16 0, Variant=w539) -> (data=w537:u16)  [unwired: 1 in, 1 out]
          n311 = Select "Use Default\nLocation?"(t=w513, s=w514, f=w502) -> (s? t:f=w523:path)
          n312 = Number To Fractional String(number=w537, precision (6)=i16 0) -> (F-format string=w550:string)  [unwired: 2 in]
          n313 = Number To Fractional String(number=w541, precision (6)=i16 0) -> (F-format string=w552:string)  [unwired: 2 in]
          n314 = Select(t="YES", s=w533, f="NO") -> (s? t:f=w554:string)
          n315 = Replace Array Subset "Update\nTest Detail\nCells"(array=w490, new element #1=w590, index (row) #1=w596, index (col) #1=w593, new element #2=w552, index (row) #2=w595, index (col) #2=w593, new element #3=w554, index (row) #3=w597, index (col) #3=w593, new element #4=w550, index (row) #4=w594, index (col) #4=w593) -> (w548:string[][])
          n316 = property on="New Test Name" class="Str"(reference=w530, "Visible"=FALSE) -> ()  [unwired: 1 in, 2 out]
          n317 = Array Subset "Details\nOnly"(array=w548, length (row)=w549) -> (w547:string[][])  [unwired: 3 in]
          n318 = Matrix Size(0:w479) -> (2:w480:i32)  [unwired: 1 out]
          n319 = Initialize Array "Blank\nCustom Row (Indexes)"(0 ("32bit integer"), w480) -> (w478:i32[])
          n320 = for "Index by Test Steps" {
            tunnel: [w605] -> w491 mode=indexing
            tunnel: w482 -> [w609] mode=indexing
            tunnel: w478 -> [w608]
            n321 = Unbundle By Name(w609) -> ("Custom Actions"=w612:u16, "ch0"=w611:bool)
            n322 = Boolean To (0,1)(Boolean=w611) -> (0, 1=w610:i16)
            n323 = To Long Integer(number=w612) -> (32bit integer=w607:i32)
            n324 = To Long Integer(number=w610) -> (32bit integer=w606:i32)
            n325 = Replace Array Subset "Insert\nValues"(array=w608, new element #1=w607, new element #2=w606) -> (w605:i32[])  [unwired: 2 in]
          }
          n326 = for "Index Test Steps" {
            tunnel: w491 -> [w600] mode=indexing
            tunnel: w479 -> [w599]
            tunnel: [w598] -> w487 mode=indexing
            n327 = for "Index Parameters" {
              tunnel: w600 -> [w604] mode=indexing
              tunnel: w599 -> [w601]
              tunnel: [w603] -> w598 mode=indexing
              i -> [w602]
              n328 = Index Array "Select\nOption"(array=w601, index (row)=w604, index (col)=w602) -> (element=w603:string)
            }
          }
          n329 = Insert Into Array "Combine\nStandard\nand Custom\nTest Values"(array=w486, index (col)=5 ("disabled index (col)"), new element=w487) -> (w546:string[][])  [unwired: 1 in]
          n330 = Insert Into Array "Combine\nDetails and\nNew Test Values"(array=w547, new element=w546) -> (w545:string[][])  [unwired: 2 in]
          n331 = Array To Spreadsheet String "Array To \nSpreadsheet String"(delimiter (Tab)="\t" ("delimiter (\\t)"), array=w545, 3:"%s" ("format (%s)")) -> (spreadsheet string=w564:string)
          n332 = Write to Text File ("Write to\nText File")(file (use dialog)=w561, text=w564, error in=w560) -> (refnum out=w563:refnum<file>, error out=w562:errorcluster)  [unwired: 1 in, 1 out]
          n333 = Close File(refnum=w563, error in=w562) -> (error out=w543:errorcluster)  [unwired: 1 out]
          n334 = case shown="No Error" w543 {
            selector: w543 -> [w618 w627]
            tunnel: w559 -> [w626 _]
            tunnel: w532 -> [w619 _]
            tunnel: [w618 w627] -> w505
            frame No Error {
              w624 = "\r\n"
              w622 = "\""
              n335 = Concatenate Strings(w624, w624) -> (w620:string)
              n336 = Concatenate Strings("Test Sequence:", w620, w622, w619, w622, w620, "Was Saved Successfully to the Test Folder:", w620, w626, w620) -> (w625:string)
              n337 = One Button Dialog "Display\nSave Info"(message=w625) -> ()  [unwired: 1 in, 1 out]
            }
            frame Error {
            }
          }
          n338 = List Folder "List Files\nin Folder"(path=w523, pattern="*.txt", error in=w505) -> (filenames=w525:string[], error out=w503:errorcluster)  [unwired: 3 out]
          n339 = for "Remove Extension" {
            tunnel: w525 -> [w616] mode=indexing
            tunnel: ".txt" ("pattern") -> [w617]
            tunnel: [w615] -> w506 mode=indexing
            tunnel: [w613] -> w511 mode=indexing
            n340 = Search and Replace String(replace all?=TRUE ("replace all? (F)"), input string=w616, search string=w617) -> (result string=w615:string, number of replacements=w613:i32)  [unwired: 5 in, 2 out]
          }
          n341 = Add Array Elements(numeric array=w511) -> (sum=w510:i32)
          n342 = Equal To 0?(x=w510) -> (x = 0?=w509:bool)
          n343 = Select(t=string[] ["No Tests Found"], s=w509, f=w506) -> (s? t:f=w508:string[])
          n344 = property on="Load Test Ring" class="Ring"(reference=w526, "DisabledEnum"=T4."Enabled" ("Disabled"), "Strings []"=w508) -> ()  [unwired: 1 in, 2 out]
        }
      }
    }
  }
  n345 = case shown="No Error" w7 {
    selector: w7 -> [_ w861]
    tunnel: w6 -> [w650 _]
    tunnel: [errorcluster {"status"=FALSE, "code"=0, "source"=""} ("error IO") w861] -> w35
    tunnel: w24 -> [w663 _]
    tunnel: w25 -> [w662 _]
    tunnel: w26 -> [w661 _]
    tunnel: "NEXT STEP" -> [w660 _]
    tunnel: "HOLD STEP" -> [w659 _]
    tunnel: string[][] [[" seconds", "1"], [" minutes", "60"], [" hours", "3600"]] ("appended array") -> [w658 _]
    tunnel: "START TEST" -> [w649 _]
    tunnel: "STOP TEST" -> [w657 _]
    tunnel: [w656 w860] -> w9
    tunnel: [w655 w859] -> w14
    tunnel: [w654 w859] -> w13
    tunnel: [w653 w858] -> w12
    tunnel: [w652 w858] -> w11
    tunnel: [w651 "TEST ERROR"] -> w10
    frame No Error {
      w667 = "\r"
      # "Test Display:\nMode:\nStep Description:\nStep Time:\nStep 1 of 100   Loop 1 of 100"
      # "Step End Actions:\n0:  Go to Next Step\n1:  Loop to Step 0\n2:  Loop to Step N\n3:  Stop Test Mode\n4:  Stop Program"
      n346 = Array Size(array=w650) -> (size(s)=w646:i32)
      n347 = Greater Than 0?(x=w646) -> (x > 0?=w648:bool)
      n348 = And(x=w649, y=w648) -> (x .and. y?=w647:bool)
      n349 = First Call? "First\nCall?"() -> (First Call?: T/F=w668:bool)
      n350 = for {
        N: 1 -> [_]
        tunnel: w660 -> [w692]
        tunnel: [w716] -> w675
        tunnel: w657 -> [w694]
        tunnel: w659 -> [w688]
        tunnel: [w718] -> w672
        tunnel: [w717] -> w670
        tunnel: [w714] -> w676
        tunnel: [w710] -> w673
        shift-right: [w712] -> w655
        shift-left: _ -> [w703]
        shift-right: [w711] -> w654
        shift-left: _ -> [w709]
        shift-right: [w713] -> w652
        shift-left: _ -> [w690]
        tunnel: w661 -> [w708]
        tunnel: w662 -> [w707]
        tunnel: w663 -> [w706]
        tunnel: w650 -> [w701]
        tunnel: w658 -> [w704]
        tunnel: [w715] -> w666
        shift-right: [w698] -> _
        shift-left: _ -> [w686]
        tunnel: [w697] -> w656
        tunnel: w668 -> [w687]
        tunnel: u16 0 ("t") -> [w696]
        tunnel: w647 -> [w684]
        tunnel: w646 -> [w683]
        n351 = Select(t=w696, s=w687, f=w703) -> (s? t:f=w700:u16)
        n352 = Select(t=w696, s=w687, f=w709) -> (s? t:f=w705:u16)
        n353 = feedback-in #8(w692) -> ()
        n354 = feedback #8() -> (w693:bool)  [unwired: 1 in]
        n355 = To Long Integer(number=w700) -> (32bit integer=w702:i32)
        n356 = To Unsigned Word Integer(number=w683) -> (unsigned 16bit integer=w685:u16)
        n357 = Greater? "Pulse on\nTRUE"(x=w692, y=w693) -> (0:w691:bool)
        n358 = Index Array "Index\nTest Array"(array=w701, index=w702) -> (element=w699:T8)
        n359 = Compound Arithmetic op=OR "Stop\nTest?"(w694, w686, w687) -> (w695:bool)
        n360 = while "Boolean Latch Function" {
          tunnel: w684 -> [w723]
          shift-right: [w721] -> w697
          shift-left: _ -> [w722]
          tunnel: w695 -> [w719]
          stop <- FALSE continue-if-true
          n361 = Exclusive Or(1:w719, 2:w723) -> (0:w724:bool)
          n362 = Select(t=w723, s=w724, f=w722) -> (s? t:f=w721:bool)
        }
        n363 = Compound Arithmetic op=OR "Reset\nTimer?"(w687, w690, w688) -> (w689:bool)
        n364 = case "Test Running?" shown="True" w697 {
          tunnel: ["Mode: OFF  (Press Start to Begin)" w796] -> w710
          tunnel: w700 -> [_ w734]
          tunnel: [w727 w797] -> w715
          tunnel: w688 -> [_ w765]
          tunnel: [w730 w799] -> w712
          tunnel: [w728 w743] -> w713
          tunnel: [w729 w798] -> w711
          tunnel: w705 -> [_ w733]
          tunnel: w706 -> [_ w747]
          tunnel: [w725 w793] -> w718
          tunnel: [w725 w768] -> w717
          tunnel: [w725 w791] -> w714
          tunnel: [w725 w774] -> w716
          tunnel: w691 -> [_ w766]
          tunnel: w707 -> [_ w790]
          tunnel: w704 -> [_ w789]
          tunnel: w708 -> [_ w746]
          tunnel: w685 -> [_ w749]
          tunnel: w699 -> [_ w742]
          tunnel: [w726 w775] -> w698
          tunnel: w689 -> [_ w755]
          frame False {
            w726 = FALSE  # Stop Test Mode
            w725 = ""  # Empty
            w727 = FALSE  # Stop Program
            w728 = TRUE  # Step Complete Signal
            w729 = u16 0  # Loop Count
            w730 = u16 0  # Test Step
          }
          frame True {
            w737 = " / " ("string")
            w770 = ""  # Empty
            w778 = ""  # Empty
            w751 = i16 1 ("width (-)")
            n365 = Decrement "Last Step"(x=w749) -> (x-1=w744:u16)
            n366 = Number To Fractional String(number=w733, precision (6)=i16 0 ("width (-)")) -> (F-format string=w732:string)  [unwired: 2 out]
            n367 = Unbundle By Name(w742) -> ("Step Description"=w774:string)
            n368 = Unbundle By Name(w742) -> ("Step Time Unit"=w753:u16, "Step Time Target"=w752:dbl)
            n369 = Unbundle By Name(w742) -> ("Step End Action"=w745:u16)
            n370 = Tick Count (ms)() -> (millisecond timer value=w761:u32)
            n371 = Number To Fractional String(number=w734, precision (6)=i16 0 ("width (-)")) -> (F-format string=w735:string)  [unwired: 2 out]
            n372 = feedback #9() -> (w763:u32)  [unwired: 1 in]
            n373 = feedback #10() -> (w760:u32)  [unwired: 1 in]
            n374 = feedback-in #10(w761) -> ()
            n375 = To Long Integer(number=w753) -> (32bit integer=w784:i32)
            n376 = Index Array(array=w789, index (row) #1=w784, index (col) #1=0 ("disabled index (col)"), index (row) #2=w784, index (col) #2=1 ("index (col)")) -> (element #1=w739:string, element #2=w782:string)
            n377 = Subtract(x=w761, y=w760) -> (x-y=w756:u32)
            n378 = Add(x=w763, y=w756) -> (x+y=w764:u32)
            n379 = Select "Reset\nTimer?"(t=u32 0 ("x+y"), s=w755, f=w764) -> (s? t:f=w762:u32)
            n380 = feedback-in #9(w762) -> ()
            n381 = To Double Precision Float(number=w762) -> (double precision float=w757:dbl)
            n382 = Divide "Elapsed\nTime [s]"(x=w757, y=1000.0) -> (x/y=w754:dbl)
            n383 = Fract/Exp String To Number "Get Unit\nMultiplier"(string=w782) -> (number=w781:dbl)  [unwired: 3 in, 1 out]
            n384 = Divide(x=w754, y=w781) -> (x/y=w783:dbl)
            n385 = Multiply "Time Target\n(seconds)"(x=w752, y=w781) -> (x*y=w776:dbl)
            n386 = Number To Fractional String(number=w744, precision (6)=i16 0 ("width (-)")) -> (F-format string=w748:string)  [unwired: 2 out]
            n387 = Number To Fractional String(number=w747, precision (6)=i16 0 ("width (-)")) -> (F-format string=w736:string)  [unwired: 2 out]
            n388 = Greater Or Equal? "Step Time\nElapsed?"(x=w754, y=w776) -> (x >= y?=w750:bool)
            n389 = Or "Step\nComplete?"(x=w750, y=w766) -> (x .or. y?=w743:bool)
            n390 = case shown="True" w743 {
              tunnel: [w803 w814] -> w799
              tunnel: [w802 w813] -> w798
              tunnel: [w801 w812] -> w797
              tunnel: w790 -> [_ w811]
              tunnel: w733 -> [w802 w810]
              tunnel: [w800 w809] -> w775
              tunnel: w734 -> [w803 w808]
              tunnel: w745 -> [_ w807]
              tunnel: w747 -> [_ w806]
              tunnel: w746 -> [_ w805]
              tunnel: w744 -> [_ w804]
              frame False {
                w801 = FALSE  # Stop Program
                w800 = FALSE  # Stop Test Mode
                # "Continue With Current Step"
              }
              frame True {
                n391 = case "Step End Actions" shown="1" w807 {
                  tunnel: [w819 w828 w843 w852 w855] -> w814
                  tunnel: [w818 w834 w848 w849 w856] -> w812
                  tunnel: [w820 w821 w838 w850 w853] -> w813
                  tunnel: w808 -> [w817 w830 w844 _ _]
                  tunnel: w810 -> [w820 w822 w837 w850 w853]
                  tunnel: [w815 w831 w845 w851 w854] -> w809
                  tunnel: w811 -> [_ _ w835 _ _]
                  tunnel: w806 -> [_ w833 w847 _ _]
                  tunnel: w805 -> [_ w826 w841 _ _]
                  tunnel: w804 -> [w816 _ _ _ _]
                  frame 0, Default {
                    w818 = FALSE  # Stop Program
                    # "Continue to Next\nTest Step"
                    n392 = Equal? "Last\nStep?"(x=w817, y=w816) -> (x = y?=w815:bool)
                    n393 = Increment(x=w817) -> (x+1=w819:u16)
                  }
                  frame 1 {
                    w832 = FALSE  # Stop Test?
                    w834 = FALSE  # Stop Program
                    w829 = u16 0  # Step #
                    # "Loop to\nTest Step 0"
                    n394 = Greater Or Equal? "Loop\nLimit?"(x=w822, y=w833) -> (x >= y?=w825:bool)
                    n395 = Increment(x=w830) -> (x+1=w827:u16)
                    n396 = Increment(x=w822) -> (x+1=w823:u16)
                    n397 = And(x=w826, y=w825) -> (x .and. y?=w824:bool)
                    n398 = Select(t=w832, s=w826, f=w825) -> (s? t:f=w831:bool)
                    n399 = Select "Next Step?"(t=w827, s=w824, f=w829) -> (s? t:f=w828:u16)
                    n400 = Select(t=w822, s=w824, f=w823) -> (s? t:f=w821:u16)
                  }
                  frame 2 {
                    w846 = FALSE  # Stop Test?
                    w848 = FALSE  # Stop Program
                    # "Loop to\nTest Step N"
                    n401 = Greater Or Equal? "Loop\nLimit?"(x=w837, y=w847) -> (x >= y?=w840:bool)
                    n402 = Increment(x=w844) -> (x+1=w842:u16)
                    n403 = Increment(x=w837) -> (x+1=w839:u16)
                    n404 = And(x=w841, y=w840) -> (x .and. y?=w836:bool)
                    n405 = Select(t=w846, s=w841, f=w840) -> (s? t:f=w845:bool)
                    n406 = Select "Next Step?"(t=w842, s=w836, f=w835) -> (s? t:f=w843:u16)
                    n407 = Select(t=w837, s=w836, f=w839) -> (s? t:f=w838:u16)
                  }
                  frame 3 {
                    w849 = FALSE  # Stop Program
                    w851 = TRUE  # Stop Test Mode
                    w852 = u16 0  # Step #
                    # "De-Activate \nTest Mode"
                  }
                  frame 4 {
                    w854 = FALSE  # Stop Test Mode
                    w855 = u16 0  # Step #
                    w856 = TRUE  # Stop Program
                    # "Stop Entire\nLabVIEW Program"
                  }
                }
              }
            }
            n408 = Equal To 0? "No Loops?"(x=w747) -> (x = 0?=w767:bool)
            n409 = Number To Fractional String "Time\nTarget"(number=w752, precision (6)=w751) -> (F-format string=w740:string)  [unwired: 2 out]
            n410 = Number To Fractional String "Time \nElapsed"(number=w783, precision (6)=w751) -> (F-format string=w787:string)  [unwired: 2 out]
            n411 = Concatenate Strings("Step: ", w735, w737, w748) -> (w793:string)
            n412 = Concatenate Strings("Loop: ", w732, w737, w736) -> (w769:string)
            n413 = Concatenate Strings("Time: ", w787, " of ", w740, w739, "." ("string")) -> (w777:string)
            n414 = Select "Hide\nLoop Text?"(t=w770, s=w767, f=w769) -> (s? t:f=w768:string)
            n415 = Select "Hold\nStep?"(t="Mode: HOLD", s=w765, f="Mode: RUN") -> (s? t:f=w796:string)
            n416 = Select(t=w778, s=w765, f=w777) -> (s? t:f=w791:string)
          }
        }
      }
      n417 = First Call?() -> (First Call?: T/F=w665:bool)
      n418 = while "Boolean Latch Function" {
        tunnel: w666 -> [w681]
        shift-right: [w679] -> w653
        shift-left: _ -> [w680]
        tunnel: w665 -> [w677]
        stop <- FALSE continue-if-true
        n419 = Exclusive Or(1:w677, 2:w681) -> (0:w682:bool)
        n420 = Select(t=w681, s=w682, f=w680) -> (s? t:f=w679:bool)
      }
      n421 = Concatenate Strings(w673, w667, w675, w667, w676, w667, w672, "    " ("String"), w670) -> (w651:string)
    }
    frame Error {
      w858 = FALSE ("Stop Program")
      w859 = u16 0 ("Step #")
      w860 = FALSE  # Test Not Active if Error Present
    }
  }
  "Error Output" <- w35
  "Step Number" <- w14
  "Loop Number" <- w13
  "Stop Program?" <- w12
  "Step Complete?" <- w11
  "Test Display" <- w10
  "Test Running?" <- w9
  n422 = feedback-in #1(w9) -> ()
  n423 = Exclusive Or "State Change?"(1:w30, 2:w9) -> (0:w29:bool)
  n424 = Or(x=w29, y=w27) -> (x .or. y?=w28:bool)
  n425 = case "Disable Controls when Test is Running" shown="True" w28 {
    tunnel: w66 -> [_ w880]
    tunnel: w9 -> [_ w862]
    tunnel: w65 -> [_ w875]
    tunnel: w27 -> [_ w864]
    frame False {
    }
    frame True {
      n426 = Unbundle By Name(w880) -> ("Save Test"=w879:i32, "Erase Test"=w878:i32, "Test Description"=w874:i32, "Load Test Ring"=w873:i32, "Test Array (Standard)"=w872:i32, "Test Array (Custom)"=w871:i32)
      n427 = Select(t=FALSE, s=w864, f=w862) -> (s? t:f=w863:bool)
      n428 = Select(t=T4."Disabled" ("Disabled"), s=w863, f=T4."Enabled" ("Disabled")) -> (s? t:f=w866:T4)
      n429 = Index Array(array=w875, index #1=w879, index #2=w878, index #3=w874, index #4=w873, index #5=w872, index #6=w871) -> (element #1=w877:refnum<vi>, element #2=w876:refnum<vi>, element #3=w870:refnum<vi>, element #4=w869:refnum<vi>, element #5=w868:refnum<vi>, element #6=w867:refnum<vi>)
      n430 = property class="Ctl"(reference=w877, "DisabledEnum"=w866) -> ()  [unwired: 1 in, 2 out]
      n431 = property class="Ctl"(reference=w876, "DisabledEnum"=w866) -> ()  [unwired: 1 in, 2 out]
      n432 = property class="Ctl"(reference=w870, "DisabledEnum"=w866) -> ()  [unwired: 1 in, 2 out]
      n433 = property class="Ctl"(reference=w869, "DisabledEnum"=w866) -> ()  [unwired: 1 in, 2 out]
      n434 = property class="Ctl"(reference=w868, "DisabledEnum"=w866) -> ()  [unwired: 1 in, 2 out]
      n435 = property class="Ctl"(reference=w867, "DisabledEnum"=w866) -> ()  [unwired: 1 in, 2 out]
    }
  }
  n436 = Unbundle By Name("Test Cluster") -> ("Test Array (Custom)"=w17:T6)
  n437 = Index Array "Get\nElement"(array=w17) -> (element=w19:T1)  [unwired: 1 in]
  n438 = Initialize Array "Create\nEmpty Array"(w19, 0 ("dimension size")) -> (w18:T6)
  n439 = To Long Integer(number=w14) -> (32bit integer=w16:i32)
  n440 = Select "Test\nRunning?"(t=w17, s=w9, f=w18) -> (s? t:f=w15:T6)
  n441 = Index Array "Index Custom Array"(array=w15, index=w16) -> (element=→"Test Output":T1)
